vi "MegaAwesome_9_20_12a_JW.vi"() -> ()   [LabVIEW 2011]
uses:
  MegaAwesome_States.ctl
  <vilib>/Utility/file.llb/Read From Spreadsheet File (string).vi
  <vilib>/Utility/file.llb/Write To Spreadsheet File (string).vi
  <vilib>/Utility/inputDevices.llb/keyboardAcquire.vi
panel:
  in  "Slider Min":dbl=5.0
  in  "Slider Max":dbl=5.0
  out "Opj X Axis":string
  out "X Axis Display Type":string
  in  "Index-Sat":dbl=5.0
  in  "Index-Lin":dbl=5.0
  in  "IndexLog-Lin":dbl=5.0
  in  "IndexLog-Sat":dbl=5.0 caption="Num Pts"
  out "Lin Id-Log Used":dbl[](array[numeric])
  out "Lin-Vg Array-Log Used":dbl[](array[numeric])
  in  "New: Comments":string
  out "Save Array":string[][](array[string])
  out "Folder Index":i32 caption="Length"
  out "Sat Id-Used":dbl[](array[numeric])
  out "Sat Vg Array-Used":dbl[](array[numeric])
  out "Vg Array-Log-Used":dbl[](array[numeric])
  out "Sat Id-Log-Used":dbl[](array[numeric])
  out "Lin Id-Used":dbl[](array[numeric])
  out "Lin-Vg Array-Used":dbl[](array[numeric])
  out "Lin Vd":dbl
  out "Recorded Prop":T1
  out "Current State":T2
  in  "Main Tab Control":T3(tab)
  in  "Image Folder":path
  out "Image File":path=path "D:/UserData/Desktop/Jeremy/WFU/Research/Programs/VI mods/Image Not Found.png"
  in  "Transfer File":path
  out "Transfer Folder":path
  out "Fabrication Prop":T4
  in  "Transport ?":bool
  out "Distances":dbl[](array[numeric])
  in  "Zoom":i16(slide)=-3 scale=-5.0..5.0
  in  "Magnification":u16(ring) items=["5x", "10x", "20x", "50x", "80x"]
  in  "Undo Button":bool
  in  "Remove Button":bool
  in  "Transfer Plots":T5(tab)=enum."Saturation"
  in  "Lin-Trans Slider":dbl(slide) step=1.0 scale=-40.0..40.0 scale format="%#_1p"
  out "Sqrt-Lin":cluster{dbl[], dbl[]}[](graph)
  in  "Sat-Trans Slider":dbl(slide) step=1.0 scale=-40.0..40.0 scale format="%#_1p"
  out "Sqrt-Sat":cluster{dbl[], dbl[]}[](graph)
  out "Raw- Lin":cluster{dbl[], dbl[]}[](graph)
  out "Raw- Sat":cluster{dbl[], dbl[]}[](graph)
  in  "Log Plots":enum32{"Linear", "Saturation", "Transport"}(tab)=enum."Saturation"
  in  "Lin-Log Slider":dbl(slide) step=1.0 scale=-40.0..40.0 scale format="%#_1p"
  out "Log-Lin":cluster{dbl[], dbl[]}[](graph)
  in  "Sat-Log Slider":dbl(slide) step=1.0 scale=-40.0..40.0 scale format="%#_1p"
  out "Sat-Log":cluster{dbl[], dbl[]}[](graph)
  out "Transport":cluster{dbl[], dbl[]}[](graph)
  in  "Manual Controls":T6
  in  "File Controls":T7
  out "Date Recorded":string="Date Recorded" caption="Measured"
  out "Data Name:":string
  out "Image Name":string
  out "Index":string
  out "Date Created":string caption="Fabricated"
  in  "Comments:":string
  out "Rec: Length":dbl caption="Length" format="%#_3g"
  out "Rec: Width":dbl caption="Width" format="%#_4g"
  out "Rec: Dielectric (d)":dbl caption="Dielectric (d)" format="%#_3g"
  in  "New: Dielectric":dbl
  in  "New: Length":dbl
  in  "New: Width":dbl
  out "Rec: Temp":dbl caption="Sample Temp" format="%.1f"
  in  "New: Temp":dbl format="%.1f"
  out "Image Out":T8(plugin-control)
  in  "Num Pts":dbl=5.0
  in  "Num Pts Log":dbl=5.0 caption="Num Pts"
  out "Recorded Values Cluster":T9
  out "Calculated Values Cluster":T9 caption="Recorded Values Cluster"
  out "Re-Calculated Values Cluster":T9 caption="Recorded Values Cluster"
  in  "Independant Variable:":string(combo)="Length (um):"
  out "Image Preview":T8(plugin-control)
  out "Total Width":dbl
  in  "No Image File":path=path "\\\\acad1\\physics/Jurchescu-group/JW-PD/Mega Awesome/Image Not Found.png"
  in  "Room Temp":dbl=294.0
  in  "Origin Project File":path=path "\\\\acad1\\physics/Jurchescu-group/JW-PD/Group Library/Origin Project Files/DeviceData_8_10_12a_JW.opj"
  in  "Transport Style Controls":T10={"Transport Line Size"=1, "Transport Line Color"=16772608} {"Transport Line Size" items=["Extra Small", "Small", "Medium", "Large", "Extra Large"]}
  # "Image Location"
  # "Recorded"
  # "Calculated"
  # "Re-Calculated"
  # "Manual"
  # "Used points display at y=0\nValues are wrong w/ slider"
  # "Slider\nDoesn't\nWork"
  # "Slider\nDoesn't\nWork"
  # "No new points displayed"
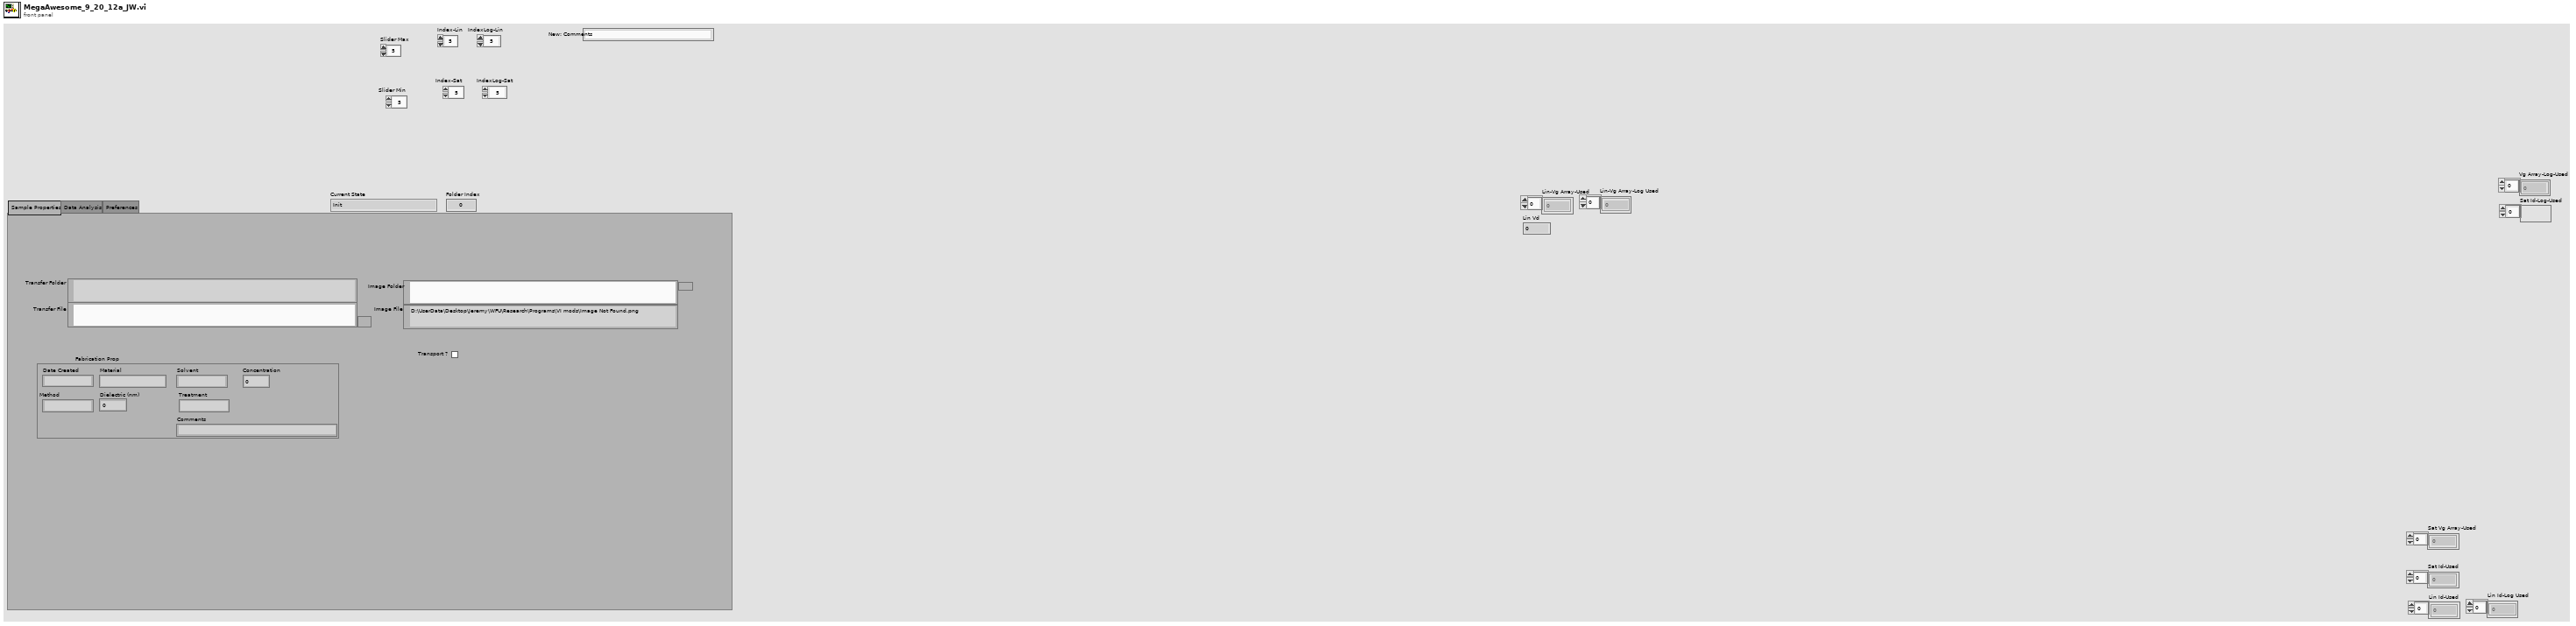
[diagram p1: front panel]
types:
  T1 = cluster{"Date Recorded":string, "Index":string, "Length":dbl, "Width":dbl, "Sample Temp":dbl}
  T2 = typedef "MegaAwesome_States.ctl" = enum16{"Init", "File Missing", "No Event", "Read Data", "Calculated Values", "Re-Calculated Values", "Next File", "Previous File", "Discard File", "Save", "Save Lines", "Export", "Exit"}
  T3 = enum32{"Sample Properties", "Data Analysis", "Preferences"}
  T4 = cluster{"Date Created":string, "Material":string, "Solvent":string, "Concentration":dbl, "Method":string, "Dielectric (nm)":dbl, "Treatment":string, "Comments":string}
  T5 = enum32{"Linear", "Saturation", "Raw-Linear", "Raw-Saturation"}
  T6 = cluster{"Manual-Temp":bool, "Manual-Width":bool, "Manuel-Length":bool, "Manuel-Dielectric":bool, "Manual Comments":bool}
  T7 = cluster{"Previous File":bool, "Discard ":bool, "Save Lines":bool, "Close":bool, "Next File ":bool, "Save":bool, "Save Next":bool, "Export":bool}
  T8 = typedef "IMAQ Image.ctl" = refnum<image>
  T9 = cluster{"Mobility-Sat":dbl, "Moblitity-Lin":dbl, "On/Off":dbl, "Off Current":dbl, "Vt-Sat":dbl, "STS":dbl, "Trap Density-VT":dbl, "Trap Density-STS":dbl}
  T10 = cluster{"Transport Line Size":u16, "Transport Line Color":u32}
  T11 = typedef "LVBoundsTypeDef.ctl" = cluster{"Width":u32, "Height":u32}
  T12 = enum16{"0", "1", "2", "3", "4", "5", "6", "7", "8", "9", "A", "B", "C", "D", "E", "F", "G", "H", "I", "J", "K", "L", "M", "N", "O", "P", "Q", "R", "S", "T", "U", "V", "W", "X", "Y", "Z", "F1", "F2", "F3", "F4", "F5", "F6", "F7", "F8", "F9", "F10", "F11", "F12", "F13", "F14", "F15", "ADD", "BACK", "BACKSLASH", "CAPITAL", "COMMA", "DECIMAL", "DELETE", "DIVIDE", "DOWN", "END", "EQUALS", "ESCAPE", "GRAVE (`)", "HOME", "INSERT", "LBRACKET", "LCONTROL", "LEFT", "L ALT", "LSHIFT", "LWIN", "MINUS", "MULTIPLY", "NEXT", "NUMLOCK", "NUMPAD_0", "NUMPAD_1", "NUMPAD_2", "NUMPAD_3", "NUMPAD_4", "NUMPAD_5", "NUMPAD_6", "NUMPAD_7", "NUMPAD_8", "NUMPAD_9", "PAUSE", "PERIOD", "PRIOR (PG UP)", "RBRACKET", "RCONTROL", "RETURN", "RIGHT", "R ALT", "RSHIFT", "RWIN", "SCROLL", "SEMICOLON", "SLASH", "SPACE", "SUBTRACT", "TAB", "UP", "ENTER (num pad)", "' (quote)"}[]
  T13 = enum16{"0", "1", "2", "3", "4", "5", "6", "7", "8", "9", "A", "B", "C", "D", "E", "F", "G", "H", "I", "J", "K", "L", "M", "N", "O", "P", "Q", "R", "S", "T", "U", "V", "W", "X", "Y", "Z", "F1", "F2", "F3", "F4", "F5", "F6", "F7", "F8", "F9", "F10", "F11", "F12", "F13", "F14", "F15", "ADD", "BACK", "BACKSLASH", "CAPITAL", "COMMA", "DECIMAL", "DELETE", "DIVIDE", "DOWN", "END", "EQUALS", "ESCAPE", "GRAVE (`)", "HOME", "INSERT", "LBRACKET", "LCONTROL", "LEFT", "L ALT", "LSHIFT", "LWIN", "MINUS", "MULTIPLY", "NEXT", "NUMLOCK", "NUMPAD_0", "NUMPAD_1", "NUMPAD_2", "NUMPAD_3", "NUMPAD_4", "NUMPAD_5", "NUMPAD_6", "NUMPAD_7", "NUMPAD_8", "NUMPAD_9", "PAUSE", "PERIOD", "PRIOR (PG UP)", "RBRACKET", "RCONTROL", "RETURN", "RIGHT", "R ALT", "RSHIFT", "RWIN", "SCROLL", "SEMICOLON", "SLASH", "SPACE", "SUBTRACT", "TAB", "UP", "ENTER (num pad)", "' (quote)"}
  T14 = typedef "ROI Descriptor" = cluster{"Global Rectangle":i32[], "Contours":cluster{"ID":enum32{"External", "Internal"}, "Type":u32, "Coordinates":i32[]}[]}
  T15 = cluster{string, sgl, bool, bool, bool, bool, bool, bool, i32}
  T16 = cluster{"[0]":cluster{dbl[], dbl[]}, "[1]":cluster{dbl[], dbl[]}, "[2]":cluster{dbl[], dbl[]}, "[3]":cluster{dbl[], dbl[]}, "[4]":cluster{dbl[], dbl[]}, "[5]":cluster{dbl[], dbl[]}, "[6]":cluster{dbl[], dbl[]}, "[7]":cluster{dbl[], dbl[]}, "[8]":cluster{dbl[], dbl[]}}
  T17 = cluster{"Sat Vg Used":dbl[], "Sat Sqrt(Id) Used ":dbl[], "Lin Vg Used":dbl[], "Lin Sqrt(Id) Used":dbl[], "Index-Lin":dbl, "Index-Sat":dbl}
  T18 = cluster{"Raw Sat":cluster{dbl[], dbl[]}[], "Sqrt Sat":cluster{dbl[], dbl[]}[], "Log Sat":cluster{dbl[], dbl[]}[], "Raw Lin":cluster{dbl[], dbl[]}[], "Sqrt Lin":cluster{dbl[], dbl[]}[], "Log Lin":cluster{dbl[], dbl[]}[]}
  T19 = cluster{"Mobility-Sat":dbl, "Vt-Sat":dbl, "Mobility-Lin":dbl, "Vt-Lin":dbl, "Off I-Sat":dbl, "On/Off I-Sat":dbl}
  T20 = cluster{"Sat Vg Used":dbl[], "Sat Log(Id) Used":dbl[], "Lin Vg Used":dbl[], "Lin Log(Id) Used":dbl[], "STS Index-Sat":dbl, "STS Index-Lin":dbl}
  T21 = cluster{"Independant  Variable Indicator":string, "Parameter String Indicator":string}
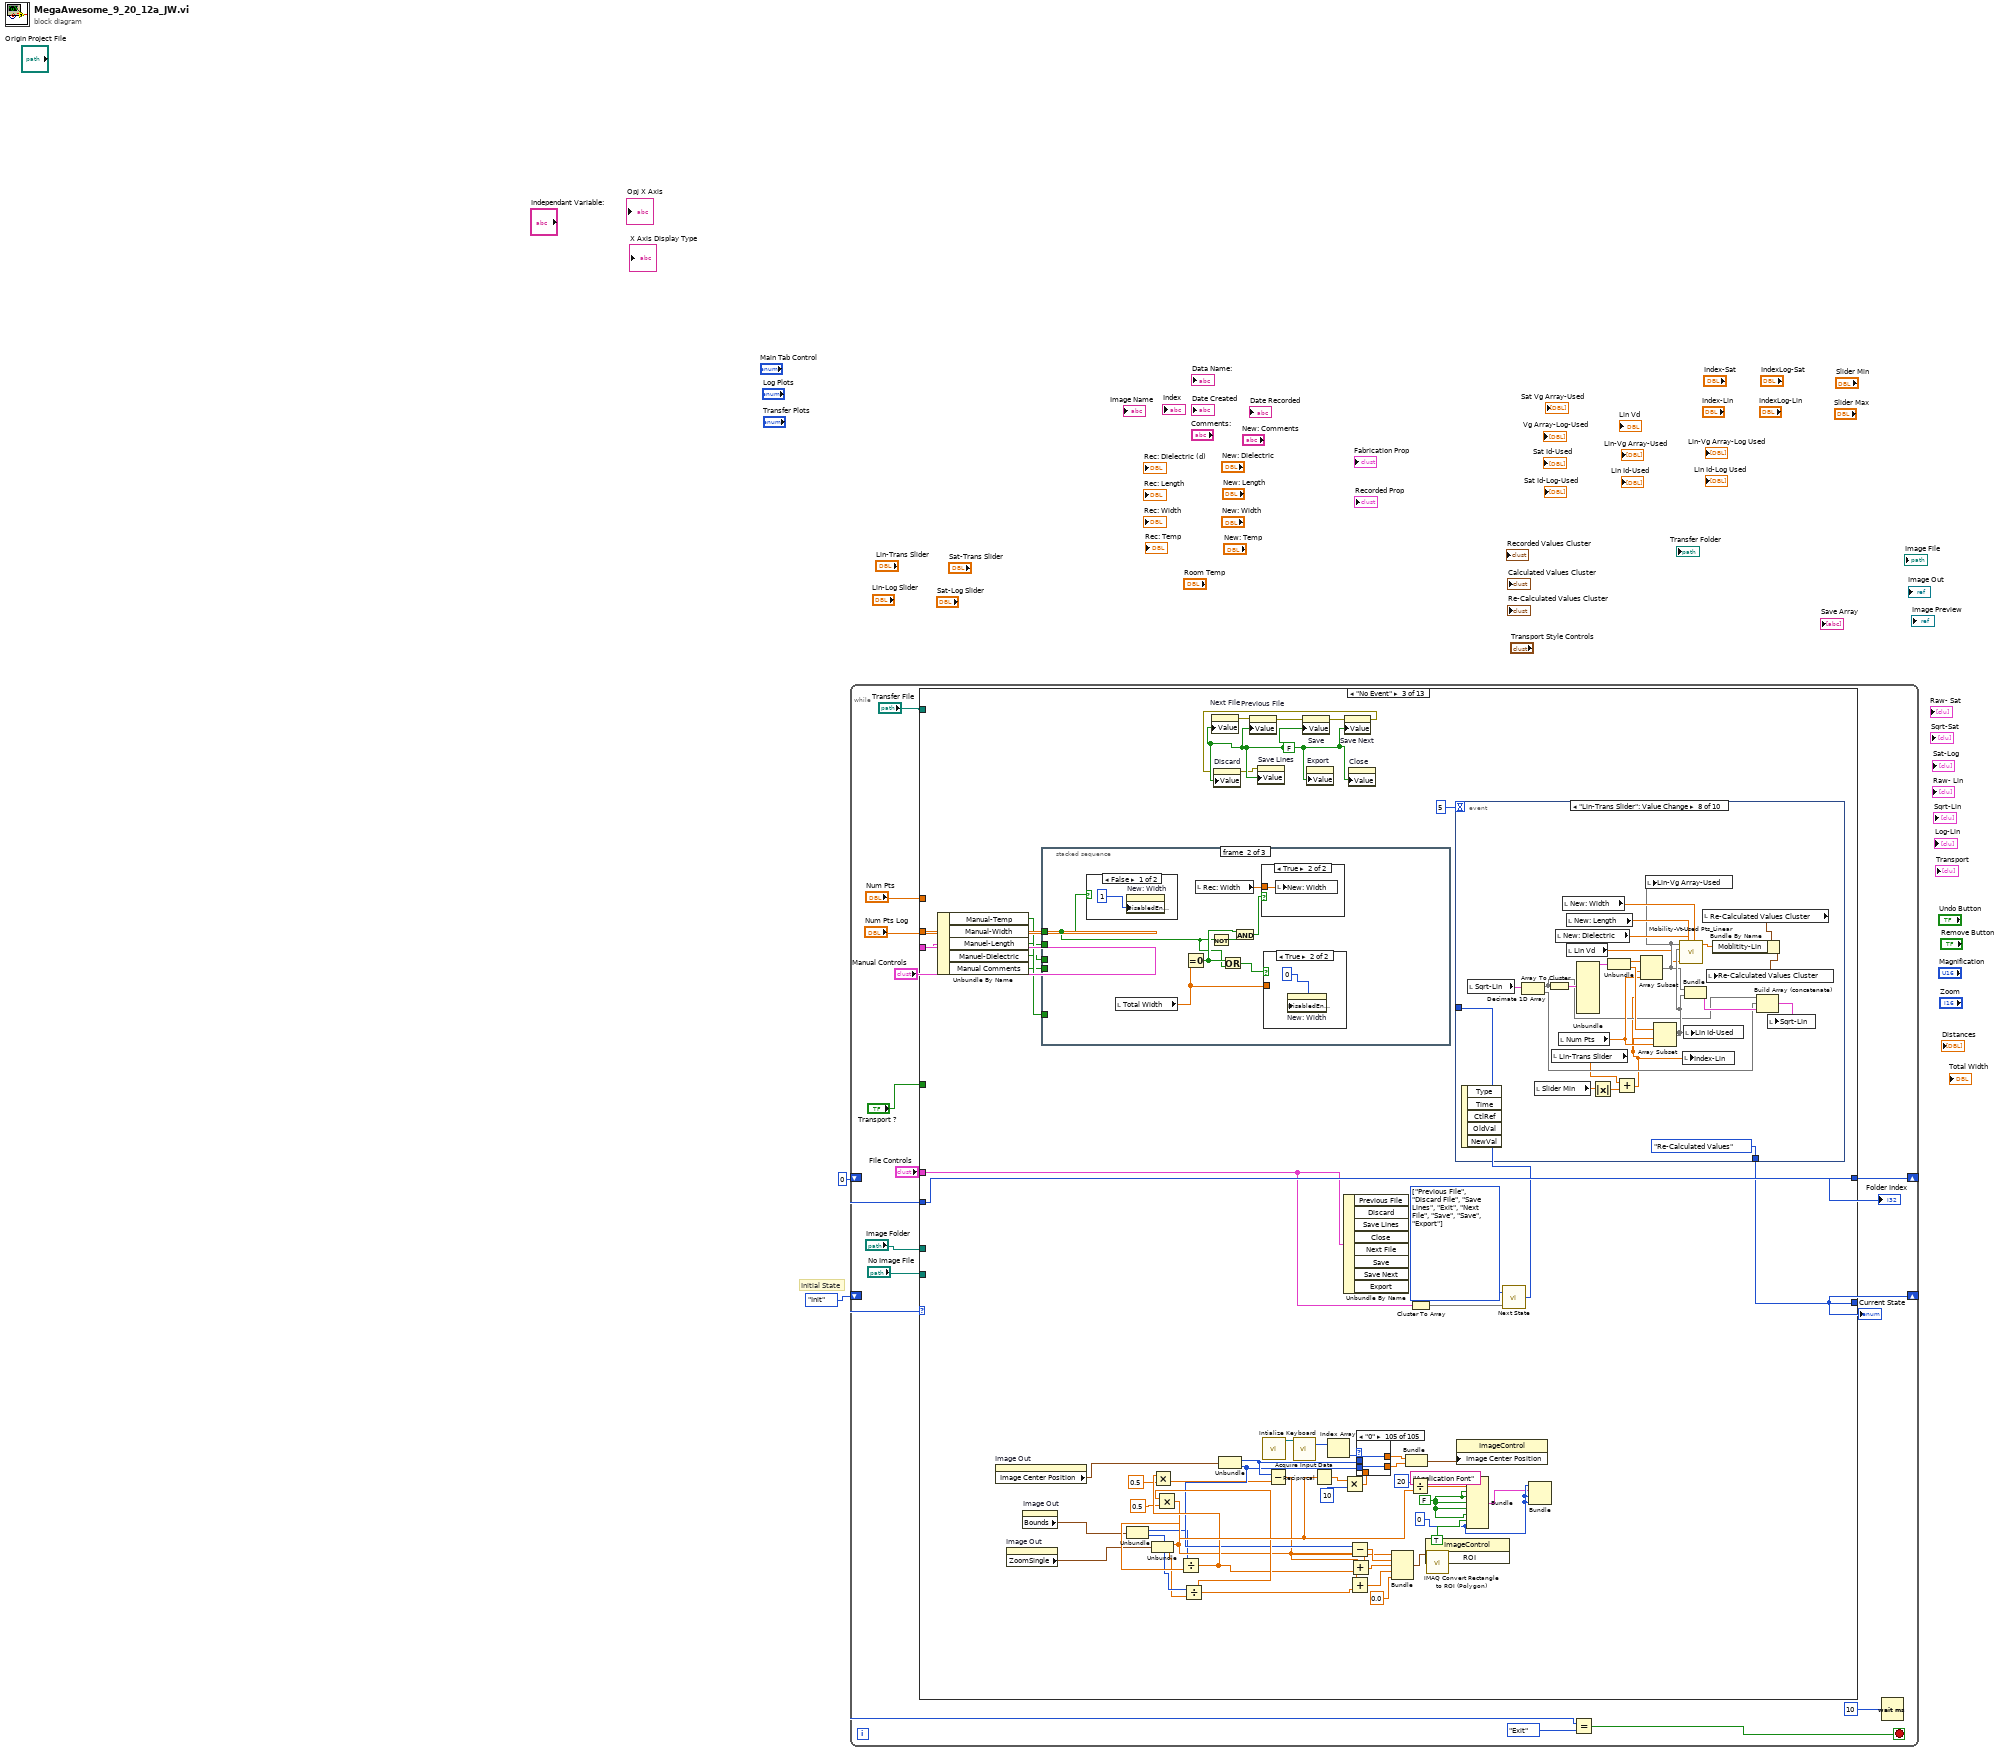
[diagram p0: block diagram]
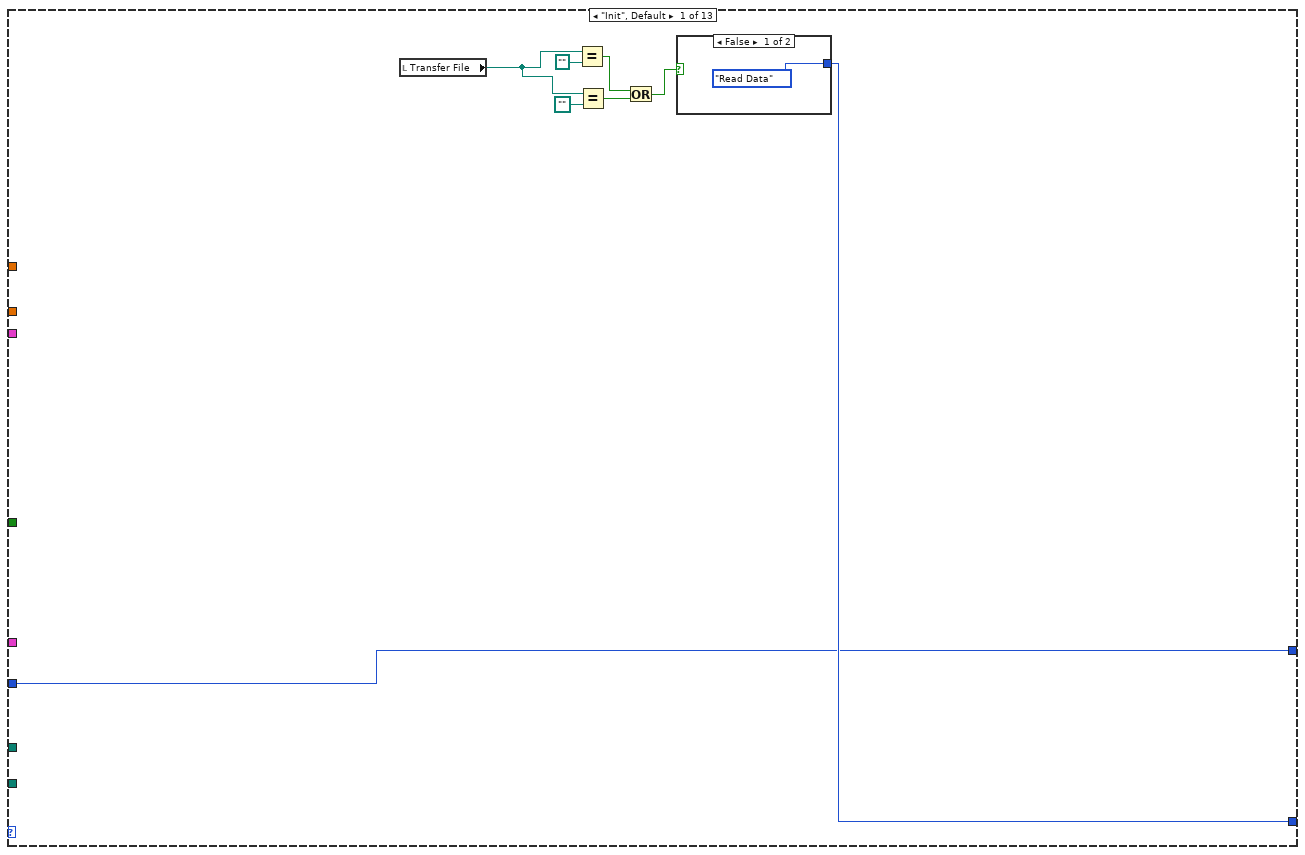
[diagram p2: hidden frame]
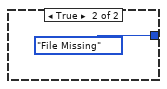
[diagram p3: hidden frame]
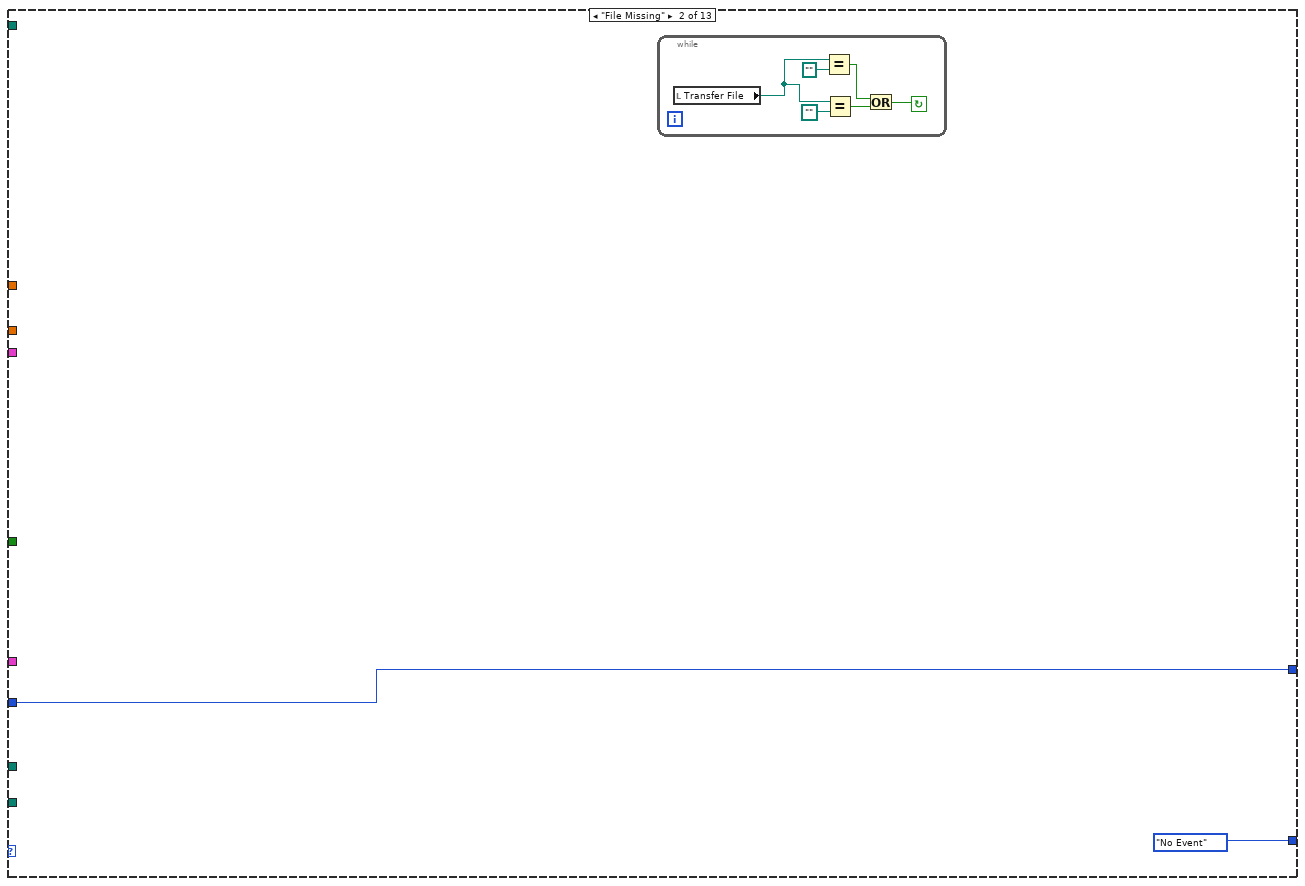
[diagram p4: hidden frame]
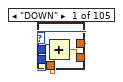
[diagram p5: hidden frame]
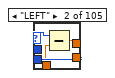
[diagram p6: hidden frame]
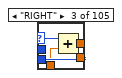
[diagram p7: hidden frame]
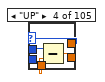
[diagram p8: hidden frame]
diagram:
  # "Initial State"
  n1 = while {
    shift-right: [w14] -> _
    shift-left: MegaAwesome_States."Init" -> [w16]
    shift-right: [w7] -> _
    shift-left: 0 -> [w8]
    stop <- w17 stop-if-true
    n2 = case shown="\"No Event\"" w16 {
      tunnel: [w19 MegaAwesome_States."No Event" w82 MegaAwesome_States."Calculated Values" MegaAwesome_States."Re-Calculated Values" MegaAwesome_States."No Event" MegaAwesome_States."Read Data" MegaAwesome_States."Read Data" MegaAwesome_States."No Event" w600 MegaAwesome_States."No Event" MegaAwesome_States."No Event" MegaAwesome_States."Exit"] -> w14
      tunnel: "Transfer File" -> [_ _ _ w445 w480 _ w569 w581 _ w605 _ _ _]
      tunnel: "Num Pts" -> [_ _ _ _ w504 _ _ _ _ _ _ _ _]
      tunnel: "Num Pts Log" -> [_ _ _ _ w503 _ _ _ _ _ _ _ _]
      tunnel: "Image Folder" -> [_ _ _ _ w500 _ _ _ _ _ _ _ _]
      tunnel: "No Image File" -> [_ _ _ _ w499 _ _ _ _ _ _ _ _]
      tunnel: [w18 w28 w90 w439 w498 w529 w554 w579 w597 w606 w1121 w1124 w1125] -> w7
      tunnel: w8 -> [w18 w28 w90 _ w498 w529 w555 w580 w597 w606 w1121 w1124 w1125]
      tunnel: "Manual Controls" -> [_ _ w84 _ _ _ _ _ _ w604 _ _ _]
      tunnel: "File Controls" -> [_ _ w80 _ _ _ _ _ _ w599 _ _ _]
      tunnel: "Transport ?" -> [_ _ _ _ w466 _ _ _ _ _ _ _ _]
      frame "Init", Default {
        n3 = local read "Transfer File"() -> (w20:path)
        n4 = Equal?(x=w20, y=path "") -> (x = y?=w23:bool)
        n5 = Equal?(x=w20, y=path "") -> (x = y?=w22:bool)
        n6 = Or(x=w23, y=w22) -> (x .or. y?=w25:bool)
        n7 = case shown="False" w25 {
          tunnel: [MegaAwesome_States."Read Data" MegaAwesome_States."File Missing"] -> w19
          frame False {
          }
          frame True {
          }
        }
      }
      frame "File Missing" {
        n8 = while {
          stop <- w30 continue-if-true
          n9 = local read "Transfer File"() -> (w31:path)
          n10 = Equal?(x=w31, y=path "") -> (x = y?=w33:bool)
          n11 = Equal?(x=w31, y=path "") -> (x = y?=w34:bool)
          n12 = Or(x=w33, y=w34) -> (x .or. y?=w30:bool)
        }
      }
      frame "No Event" {
        w64 = FALSE
        w66 = 0
        w79 = FALSE
        w92 = T2[] [enum."Previous File", enum."Discard File", enum."Save Lines", enum."Exit", enum."Next File", enum."Save", enum."Save", enum."Export"] items=["Init", "File Missing", "No Event", "Read Data", "Calculated Values", "Re-Calculated Values", "Next File", "Previous File", "Discard File", "Save", "Save Lines", "Export", "Exit"]
        n13 = Unbundle By Name(w84) -> ("Manual-Temp"=w89:bool, "Manual-Width"=w88:bool, "Manuel-Length"=w87:bool, "Manuel-Dielectric"=w86:bool, "Manual Comments"=w85:bool)
        n14 = property on="Image Out" class="ImageControl"() -> ("Image Center Position"=w42:cluster{"X":u32, "Y":u32})  [unwired: 2 in, 2 out]
        n15 = property on="Image Out" class="ImageControl"() -> ("ZoomSingle"=w49:cluster{"X":sgl, "Y":sgl})  [unwired: 2 in, 2 out]
        n16 = property on="Image Out" class="ImageControl"() -> ("Bounds"=w48:T11)  [unwired: 2 in, 2 out]
        n17 = stacked-sequence {
          tunnel: w89 -> [w403 _ _]
          tunnel: w88 -> [_ w413 _]
          tunnel: w87 -> [_ _ w428]
          tunnel: w86 -> [_ _ w425]
          tunnel: w85 -> [_ _ w424]
          frame #0 {
            n18 = local read "Rec: Temp"() -> (w402:dbl)
            n19 = case shown="False" w403 {
              tunnel: w402 -> [w408 _]
              tunnel: [w405 w412] -> _
              frame False {
                n20 = local read "Rec: Temp"() -> (w406:dbl)
                n21 = property on="New: Temp" class="DigNum (strict)"("DisabledEnum"=1) -> ()  [unwired: 2 in, 2 out]
                n22 = Equal To 0?(x=w406) -> (x = 0?=w407:bool)
                n23 = local write "New: Temp"(w408) -> ()
                n24 = case shown="True" w407 {
                  tunnel: [w409 w410] -> w405
                  tunnel: w406 -> [w409 _]
                  frame False {
                  }
                  frame True {
                    n25 = local read "Room Temp"() -> (w410:dbl)
                  }
                }
                n26 = local write "New: Temp"(w405) -> ()
              }
              frame True {
                n27 = property on="New: Temp" class="DigNum (strict)"("DisabledEnum"=0) -> ()  [unwired: 2 in, 2 out]
                n28 = local read "New: Temp"() -> (w412:dbl)
              }
            }
          }
          frame #1 {
            n29 = case shown="False" w413 {
              frame False {
                n30 = property on="New: Width" class="DigNum (strict)"("DisabledEnum"=1) -> ()  [unwired: 2 in, 2 out]
              }
              frame True {
                (unwired) 0
              }
            }
            n31 = local read "Total Width"() -> (w419:dbl)
            n32 = Equal To 0?(x=w419) -> (x = 0?=w416:bool)
            n33 = local read "Rec: Width"() -> (w417:dbl)
            n34 = Not(x=w413) -> (.not. x?=w415:bool)
            n35 = Or(x=w416, y=w413) -> (x .or. y?=w418:bool)
            n36 = And(x=w416, y=w415) -> (x .and. y?=w414:bool)
            n37 = case shown="True" w414 {
              tunnel: w417 -> [_ w421]
              frame False {
              }
              frame True {
                n38 = local write "New: Width"(w421) -> ()
              }
            }
            n39 = case shown="True" w418 {
              tunnel: w419 -> [w422 _]
              frame False {
                (unwired) 1
                n40 = local write "New: Width"(w422) -> ()
              }
              frame True {
                n41 = property on="New: Width" class="DigNum (strict)"("DisabledEnum"=0) -> ()  [unwired: 2 in, 2 out]
              }
            }
          }
          frame #2 {
            n42 = local read "Rec: Length"() -> (w429:dbl)
            n43 = case shown="True" w428 {
              tunnel: w429 -> [w437 _]
              frame False {
                n44 = local write "New: Length"(w437) -> ()
                n45 = property on="New: Length" class="DigNum (strict)"("DisabledEnum"=1) -> ()  [unwired: 2 in, 2 out]
              }
              frame True {
                n46 = property on="New: Length" class="DigNum (strict)"("DisabledEnum"=0) -> ()  [unwired: 2 in, 2 out]
              }
            }
            n47 = local read "Comments:"() -> (w426:string)
            n48 = local read "Rec: Dielectric (d)"() -> (w427:dbl)
            n49 = case shown="True" w424 {
              tunnel: w426 -> [w431 _]
              frame False {
                n50 = local write "New: Comments"(w431) -> ()
                n51 = property on="New: Comments" class="Str"("DisabledEnum"=1) -> ()  [unwired: 2 in, 2 out]
              }
              frame True {
                n52 = property on="New: Comments" class="Str"("DisabledEnum"=0) -> ()  [unwired: 2 in, 2 out]
              }
            }
            n53 = case shown="True" w425 {
              tunnel: w427 -> [w434 _]
              frame False {
                n54 = local write "New: Dielectric"(w434) -> ()
                n55 = property on="New: Dielectric" class="DigNum (strict)"("DisabledEnum"=1) -> ()  [unwired: 2 in, 2 out]
              }
              frame True {
                n56 = property on="New: Dielectric" class="DigNum (strict)"("DisabledEnum"=0) -> ()  [unwired: 2 in, 2 out]
              }
            }
          }
        }
        n57 = Unbundle(w48) -> ("Width"=w51:u32, "Height"=w52:u32)
        n58 = Unbundle(w49) -> ("X"=w71:sgl, "Y"=w50:sgl)
        n59 = Divide(x=w51, y=w71) -> (x/y=w61:sgl)
        n60 = Multiply(x=w61, y=0.5) -> (x*y=w55:dbl)
        n61 = Divide(x=w52, y=w50) -> (x/y=w62:sgl)
        n62 = Multiply(x=w62, y=0.5) -> (x*y=w56:dbl)
        n63 = property on="Next File" class="Bool (strict)"("Value"=w79) -> (error out=w78:errorcluster)  [unwired: 2 in, 1 out]
        n64 = Unbundle(w42) -> ("X"=w60:u32, "Y"=w59:u32)
        n65 = property on="Previous File" class="Bool (strict)"(error in=w78, "Value"=w79) -> (error out=w77:errorcluster)  [unwired: 1 in, 1 out]
        n66 = call <vilib>:"Intialize Keyboard.vi"() -> ("device ID"=w39:refnum<k1>)  [unwired: 10 in, 1 out]
        n67 = Subtract(x=w60, y=w55) -> (x-y=w57:dbl)
        n68 = call-poly <vilib>:"Acquire Input Data.vi"("device ID"=w39) -> ("keys pressed"=w40:T12)  [unwired: 16 in, 2 out]
        n69 = property on="Save" class="Bool (strict)"(error in=w77, "Value"=w79) -> (error out=w76:errorcluster)  [unwired: 1 in, 1 out]
        n70 = property on="Export" class="Bool (strict)"("Value"=w79) -> ()  [unwired: 2 in, 2 out]
        n71 = Reciprocal(x=w71) -> (1/x=w72:sgl)
        n72 = Index Array(array=w40) -> (element=w36:T13)  [unwired: 1 in]
        n73 = Unbundle By Name(w80) -> ()  [unwired: 8 out]
        n74 = Multiply(x=w72, y=10) -> (x*y=w70:sgl)
        n75 = property on="Save Next" class="Bool (strict)"(error in=w76, "Value"=w79) -> (error out=w75:errorcluster)  [unwired: 1 in, 1 out]
        n76 = property on="Discard" class="Bool (strict)"(error in=w75, "Value"=w79) -> (error out=w74:errorcluster)  [unwired: 1 in, 1 out]
        n77 = property on="Save Lines" class="Bool (strict)"(error in=w74, "Value"=w79) -> ()  [unwired: 1 in, 2 out]
        n78 = property on="Close" class="Bool (strict)"("Value"=w79) -> ()  [unwired: 2 in, 2 out]
        n79 = Subtract(x=w59, y=w56) -> (x-y=w58:dbl)
        n80 = Add(x=w58, y=w62) -> (x+y=w44:dbl)
        n81 = Add(x=w57, y=w61) -> (x+y=w43:dbl)
        n82 = case shown="\"0\"" w36 {
          tunnel: w60 -> [w94 w100 w104 w106 w110 w112 w114 w116 w118 w120 w122 w124 w126 w128 w130 w132 w134 w136 w138 w140 w142 w144 w146 w148 w150 w152 w154 w156 w158 w160 w162 w164 w166 w168 w170 w172 w174 w176 w178 w180 w182 w184 w186 w188 w190 w192 w194 w196 w198 w200 w202 w204 w206 w208 w210 w212 w214 w216 w218 w220 w222 w224 w226 w228 w230 w232 w234 w236 w238 w240 w242 w244 w246 w248 w250 w252 w254 w256 w258 w260 w262 w264 w266 w268 w270 w272 w274 w276 w278 w280 w282 w284 w286 w288 w290 w292 w294 w296 w298 w300 w302 w304 w306 w308 w310]
          tunnel: [w94 w99 w103 w106 w110 w112 w114 w116 w118 w120 w122 w124 w126 w128 w130 w132 w134 w136 w138 w140 w142 w144 w146 w148 w150 w152 w154 w156 w158 w160 w162 w164 w166 w168 w170 w172 w174 w176 w178 w180 w182 w184 w186 w188 w190 w192 w194 w196 w198 w200 w202 w204 w206 w208 w210 w212 w214 w216 w218 w220 w222 w224 w226 w228 w230 w232 w234 w236 w238 w240 w242 w244 w246 w248 w250 w252 w254 w256 w258 w260 w262 w264 w266 w268 w270 w272 w274 w276 w278 w280 w282 w284 w286 w288 w290 w292 w294 w296 w298 w300 w302 w304 w306 w308 w310] -> w37
          tunnel: w59 -> [w96 w98 w102 w108 w109 w111 w113 w115 w117 w119 w121 w123 w125 w127 w129 w131 w133 w135 w137 w139 w141 w143 w145 w147 w149 w151 w153 w155 w157 w159 w161 w163 w165 w167 w169 w171 w173 w175 w177 w179 w181 w183 w185 w187 w189 w191 w193 w195 w197 w199 w201 w203 w205 w207 w209 w211 w213 w215 w217 w219 w221 w223 w225 w227 w229 w231 w233 w235 w237 w239 w241 w243 w245 w247 w249 w251 w253 w255 w257 w259 w261 w263 w265 w267 w269 w271 w273 w275 w277 w279 w281 w283 w285 w287 w289 w291 w293 w295 w297 w299 w301 w303 w305 w307 w309]
          tunnel: [w95 w98 w102 w107 w109 w111 w113 w115 w117 w119 w121 w123 w125 w127 w129 w131 w133 w135 w137 w139 w141 w143 w145 w147 w149 w151 w153 w155 w157 w159 w161 w163 w165 w167 w169 w171 w173 w175 w177 w179 w181 w183 w185 w187 w189 w191 w193 w195 w197 w199 w201 w203 w205 w207 w209 w211 w213 w215 w217 w219 w221 w223 w225 w227 w229 w231 w233 w235 w237 w239 w241 w243 w245 w247 w249 w251 w253 w255 w257 w259 w261 w263 w265 w267 w269 w271 w273 w275 w277 w279 w281 w283 w285 w287 w289 w291 w293 w295 w297 w299 w301 w303 w305 w307 w309] -> w38
          tunnel: w70 -> [w93 w97 w101 w105 _ _ _ _ _ _ _ _ _ _ _ _ _ _ _ _ _ _ _ _ _ _ _ _ _ _ _ _ _ _ _ _ _ _ _ _ _ _ _ _ _ _ _ _ _ _ _ _ _ _ _ _ _ _ _ _ _ _ _ _ _ _ _ _ _ _ _ _ _ _ _ _ _ _ _ _ _ _ _ _ _ _ _ _ _ _ _ _ _ _ _ _ _ _ _ _ _ _ _ _ _]
          frame "DOWN" {
            n83 = Add(x=w96, y=w93) -> (x+y=w95:sgl)
          }
          frame "LEFT" {
            n84 = Subtract(x=w100, y=w97) -> (x-y=w99:sgl)
          }
          frame "RIGHT" {
            n85 = Add(x=w104, y=w101) -> (x+y=w103:sgl)
          }
          frame "UP" {
            n86 = Subtract(x=w108, y=w105) -> (x-y=w107:sgl)
          }
          frame "ENTER (num pad)" {
          }
          frame "' (quote)" {
          }
          frame "END" {
          }
          frame "EQUALS" {
          }
          frame "ESCAPE" {
          }
          frame "GRAVE (`)" {
          }
          frame "HOME" {
          }
          frame "INSERT" {
          }
          frame "LBRACKET" {
          }
          frame "LCONTROL" {
          }
          frame "L ALT" {
          }
          frame "LSHIFT" {
          }
          frame "LWIN" {
          }
          frame "MINUS" {
          }
          frame "MULTIPLY" {
          }
          frame "NEXT" {
          }
          frame "NUMLOCK" {
          }
          frame "NUMPAD_0" {
          }
          frame "NUMPAD_1" {
          }
          frame "NUMPAD_2" {
          }
          frame "NUMPAD_3" {
          }
          frame "NUMPAD_4" {
          }
          frame "NUMPAD_5" {
          }
          frame "NUMPAD_6" {
          }
          frame "NUMPAD_7" {
          }
          frame "NUMPAD_8" {
          }
          frame "NUMPAD_9" {
          }
          frame "PAUSE" {
          }
          frame "PERIOD" {
          }
          frame "PRIOR (PG UP)" {
          }
          frame "RBRACKET" {
          }
          frame "RCONTROL" {
          }
          frame "RETURN" {
          }
          frame "R ALT" {
          }
          frame "RSHIFT" {
          }
          frame "RWIN" {
          }
          frame "SCROLL" {
          }
          frame "SEMICOLON" {
          }
          frame "SLASH" {
          }
          frame "SPACE" {
          }
          frame "SUBTRACT" {
          }
          frame "TAB" {
          }
          frame "DIVIDE" {
          }
          frame "DELETE" {
          }
          frame "DECIMAL" {
          }
          frame "COMMA" {
          }
          frame "CAPITAL" {
          }
          frame "BACKSLASH" {
          }
          frame "BACK" {
          }
          frame "ADD" {
          }
          frame "F15" {
          }
          frame "F14" {
          }
          frame "F13" {
          }
          frame "F12" {
          }
          frame "F11" {
          }
          frame "F10" {
          }
          frame "F9" {
          }
          frame "F8" {
          }
          frame "F7" {
          }
          frame "F6" {
          }
          frame "F5" {
          }
          frame "F4" {
          }
          frame "F3" {
          }
          frame "F2" {
          }
          frame "F1" {
          }
          frame "Z" {
          }
          frame "Y" {
          }
          frame "X" {
          }
          frame "W" {
          }
          frame "V" {
          }
          frame "U" {
          }
          frame "T" {
          }
          frame "S" {
          }
          frame "R" {
          }
          frame "Q" {
          }
          frame "P" {
          }
          frame "O" {
          }
          frame "N" {
          }
          frame "M" {
          }
          frame "L" {
          }
          frame "K" {
          }
          frame "J" {
          }
          frame "I" {
          }
          frame "H" {
          }
          frame "G" {
          }
          frame "F" {
          }
          frame "E" {
          }
          frame "D" {
          }
          frame "C" {
          }
          frame "B" {
          }
          frame "A" {
          }
          frame "9" {
          }
          frame "8" {
          }
          frame "7" {
          }
          frame "6" {
          }
          frame "5" {
          }
          frame "4" {
          }
          frame "3" {
          }
          frame "2" {
          }
          frame "1" {
          }
          frame "0" {
          }
        }
        n87 = Bundle(w57, w58, w43, w44, 0.0) -> (w45:cluster{dbl, dbl, dbl, dbl, dbl})  [unwired: 1 in]
        n88 = Bundle("X"=w37, "Y"=w38) -> (w41:cluster{"X":sgl, "Y":sgl})  [unwired: 1 in]
        n89 = Divide(x=20, y=w71) -> (x/y=w68:sgl)
        n90 = Cluster To Array(cluster=w80) -> (array=w91:bool[])
        n91 = call "IMAQ Convert Rectangle to ROI (Polygon)"("Rectangle"=w45) -> ("ROI Descriptor"=w47:T14)  [unwired: 7 in, 2 out]
        n92 = property on="Property Node" class="ImageControl"("ROI"=w47) -> ()  [unwired: 2 in, 2 out]
        n93 = property on="Property Node" class="ImageControl"("Image Center Position"=w41) -> ()  [unwired: 2 in, 2 out]
        n94 = Bundle("Application Font", w68, w64, w64, w64, w64, w64, TRUE, w66) -> (w63:T15)  [unwired: 1 in]
        n95 = call "Next State.vi"("Buttons []"=w91, "States []"=w92) -> ("Enum"=w83:T2)
        n96 = event shown="[7] \"Lin-Trans Slider\": Value Change" {
          selector: _ -> [_ _ _ _ _ _ _ _ _ _]
          dyn-events: _ -> [_ _ _ _ _ _ _ _ _ _]
          timeout: 5 -> [_ _ _ _ _ _ _ _ _ _]
          tunnel: w83 -> [w311 _ _ _ _ _ _ _ _ _]
          tunnel: [w311 MegaAwesome_States."Re-Calculated Values" MegaAwesome_States."Re-Calculated Values" MegaAwesome_States."Re-Calculated Values" MegaAwesome_States."Re-Calculated Values" MegaAwesome_States."Calculated Values" MegaAwesome_States."Re-Calculated Values" MegaAwesome_States."Re-Calculated Values" MegaAwesome_States."Re-Calculated Values" MegaAwesome_States."Re-Calculated Values"] -> w82
          event Timeout {
            n97 = event-data() -> ()  [unwired: 1 in, 2 out]
          }
          event "New: Dielectric": Value Change {
            n98 = event-data() -> ()  [unwired: 1 in, 5 out]
          }
          event "New: Length": Value Change {
            n99 = event-data() -> ()  [unwired: 1 in, 5 out]
          }
          event "New: Width": Value Change {
            n100 = event-data() -> ()  [unwired: 1 in, 5 out]
          }
          event "New: Temp": Value Change {
            n101 = event-data() -> ()  [unwired: 1 in, 5 out]
          }
          event "Num Pts Log", "Transport Style Controls", "Num Pts": Value Change {
            n102 = event-data() -> ()  [unwired: 1 in, 5 out]
          }
          event "Sat-Trans Slider": Value Change {
            n103 = event-data() -> ()  [unwired: 1 in, 5 out]
            n104 = local read "Sqrt-Sat"() -> (w340:cluster{dbl[], dbl[]}[])
            n105 = Decimate 1D Array(w340) -> (w324:cluster{dbl[], dbl[]}[], w325:cluster{dbl[], dbl[]}[])
            n106 = local read "Slider Min"() -> (w321:dbl)
            n107 = local read "Sat-Trans Slider"() -> (w319:dbl)
            n108 = Array To Cluster(array=w324) -> (cluster=w339:T16)
            n109 = local read "New: Dielectric"() -> (w334:dbl)
            n110 = local read "Num Pts"() -> (w317:dbl)
            n111 = local read "New: Width"() -> (w336:dbl)
            n112 = local read "New: Length"() -> (w335:dbl)
            n113 = Unbundle(w339) -> ("[0]"=w338:cluster{dbl[], dbl[]})  [unwired: 8 out]
            n114 = Absolute Value(x=w321) -> (abs(x)=w320:dbl)
            n115 = Unbundle(w338) -> (w322:dbl[], w337:dbl[])
            n116 = Add(x=w319, y=w320) -> (x+y=w318:dbl)
            n117 = Array Subset(array=w322, index=w318, length=w317) -> (w332:dbl[])
            n118 = local write "Sat Vg Array-Used"(w332) -> ()
            n119 = Array Subset(array=w337, index=w318, length=w317) -> (w333:dbl[])
            n120 = call "Mobility-Vt-Used Pts_Saturation.vi"("Width"=w336, "Length"=w335, "Dielectric (d)"=w334, "Sat Id Used"=w333, "Vg Used"=w332) -> ("Vt"=w328:dbl, "Mobility"=w329:dbl)  [unwired: 4 in, 1 out]
            n121 = local write "Index-Sat"(w318) -> ()
            n122 = local write "Sat Id-Used"(w333) -> ()
            n123 = Bundle(w332, w333) -> (w326:cluster{dbl[], dbl[]})  [unwired: 1 in]
            n124 = local read "Re-Calculated Values Cluster"() -> (w331:T9)
            n125 = Bundle By Name(cluster=w331, "Mobility-Sat"=w329, "Vt-Sat"=w328) -> (w330:T9)
            n126 = local write "Re-Calculated Values Cluster"(w330) -> ()
            n127 = Build Array (concatenate)(w324, w325, w326) -> (w323:cluster{dbl[], dbl[]}[])
            n128 = local write "Sqrt-Sat"(w323) -> ()
          }
          event "Lin-Trans Slider": Value Change {
            n129 = event-data() -> ()  [unwired: 1 in, 5 out]
            n130 = local read "Sqrt-Lin"() -> (w364:cluster{dbl[], dbl[]}[])
            n131 = Decimate 1D Array(w364) -> (w349:cluster{dbl[], dbl[]}[], w350:cluster{dbl[], dbl[]}[])
            n132 = local read "Slider Min"() -> (w346:dbl)
            n133 = Array To Cluster(array=w349) -> (cluster=w363:T16)
            n134 = local read "Lin-Trans Slider"() -> (w344:dbl)
            n135 = local read "New: Dielectric"() -> (w357:dbl)
            n136 = local read "Num Pts"() -> (w360:dbl)
            n137 = local read "New: Width"() -> (w359:dbl)
            n138 = local read "New: Length"() -> (w358:dbl)
            n139 = local read "Lin Vd"() -> (w341:dbl)
            n140 = Unbundle(w363) -> ("[0]"=w362:cluster{dbl[], dbl[]})  [unwired: 8 out]
            n141 = Absolute Value(x=w346) -> (abs(x)=w345:dbl)
            n142 = Unbundle(w362) -> (w347:dbl[], w361:dbl[])
            n143 = Add(x=w344, y=w345) -> (x+y=w343:dbl)
            n144 = Array Subset(array=w347, index=w343, length=w360) -> (w355:dbl[])
            n145 = local write "Lin-Vg Array-Used"(w355) -> ()
            n146 = Array Subset(array=w361, index=w343, length=w360) -> (w356:dbl[])
            n147 = call "Mobility-Vt-Used Pts_Linear.vi"("Width"=w359, "Length"=w358, "Vd"=w341, "Dielectric (d)"=w357, "Id Used"=w356, "Vg Used"=w355) -> ("Mobility"=w352:dbl)  [unwired: 3 in, 2 out]
            n148 = local write "Index-Lin"(w343) -> ()
            n149 = local write "Lin Id-Used"(w356) -> ()
            n150 = Bundle(w355, w356) -> (w351:cluster{dbl[], dbl[]})  [unwired: 1 in]
            n151 = local read "Re-Calculated Values Cluster"() -> (w354:T9)
            n152 = Bundle By Name(cluster=w354, "Moblitity-Lin"=w352) -> (w353:T9)
            n153 = local write "Re-Calculated Values Cluster"(w353) -> ()
            n154 = Build Array (concatenate)(w349, w350, w351) -> (w348:cluster{dbl[], dbl[]}[])
            n155 = local write "Sqrt-Lin"(w348) -> ()
          }
          event "Sat-Log Slider": Value Change {
            n156 = event-data() -> ()  [unwired: 1 in, 5 out]
            n157 = local read "Sat-Log"() -> (w367:cluster{dbl[], dbl[]}[])
            n158 = Decimate 1D Array(w367) -> (w374:cluster{dbl[], dbl[]}[], w375:cluster{dbl[], dbl[]}[])
            n159 = local read "Slider Min"() -> (w371:dbl)
            n160 = Array To Cluster(array=w374) -> (cluster=w384:T16)
            n161 = local read "Num Pts Log"() -> (w381:dbl)
            n162 = local read "Sat-Log Slider"() -> (w369:dbl)
            n163 = Unbundle(w384) -> ("[0]"=w383:cluster{dbl[], dbl[]})  [unwired: 8 out]
            n164 = Absolute Value(x=w371) -> (abs(x)=w370:dbl)
            n165 = Unbundle(w383) -> (w372:dbl[], w382:dbl[])
            n166 = Add(x=w369, y=w370) -> (x+y=w366:dbl)
            n167 = Array Subset(array=w372, index=w366, length=w381) -> (w379:dbl[])
            n168 = Array Subset(array=w382, index=w366, length=w381) -> (w380:dbl[])
            n169 = local write "Vg Array-Log-Used"(w379) -> ()
            n170 = local write "IndexLog-Sat"(w366) -> ()
            n171 = Bundle(w379, w380) -> (w365:cluster{dbl[], dbl[]})  [unwired: 1 in]
            n172 = call "STS-Used.vi"("Id Used"=w380, "Vg-Used"=w379) -> ("STS"=w376:dbl)  [unwired: 9 in]
            n173 = local write "Sat Id-Log-Used"(w380) -> ()
            n174 = local read "Re-Calculated Values Cluster"() -> (w378:T9)
            n175 = Bundle By Name(cluster=w378, "STS"=w376) -> (w377:T9)
            n176 = local write "Re-Calculated Values Cluster"(w377) -> ()
            n177 = Build Array (concatenate)(w374, w375, w365) -> (w373:cluster{dbl[], dbl[]}[])
            n178 = local write "Sat-Log"(w373) -> ()
          }
          event "Lin-Log Slider": Value Change {
            # "No Indicator for Lin-Log Slider Use"
            n179 = event-data() -> ()  [unwired: 1 in, 5 out]
            n180 = local read "Log-Lin"() -> (w388:cluster{dbl[], dbl[]}[])
            n181 = Decimate 1D Array(w388) -> (w394:cluster{dbl[], dbl[]}[], w395:cluster{dbl[], dbl[]}[])
            n182 = local read "Slider Min"() -> (w391:dbl)
            n183 = Array To Cluster(array=w394) -> (cluster=w401:T16)
            n184 = local read "Num Pts Log"() -> (w398:dbl)
            n185 = local read "Lin-Log Slider"() -> (w389:dbl)
            n186 = Unbundle(w401) -> ("[0]"=w400:cluster{dbl[], dbl[]})  [unwired: 8 out]
            n187 = Absolute Value(x=w391) -> (abs(x)=w390:dbl)
            n188 = Unbundle(w400) -> (w392:dbl[], w399:dbl[])
            n189 = Add(x=w389, y=w390) -> (x+y=w387:dbl)
            n190 = Array Subset(array=w392, index=w387, length=w398) -> (w396:dbl[])
            n191 = local write "Lin-Vg Array-Log Used"(w396) -> ()
            n192 = Array Subset(array=w399, index=w387, length=w398) -> (w397:dbl[])
            n193 = local write "IndexLog-Sat"(w387) -> ()
            n194 = Bundle(w396, w397) -> (w386:cluster{dbl[], dbl[]})  [unwired: 1 in]
            n195 = call "STS-Used.vi"("Id Used"=w397, "Vg-Used"=w396) -> ()  [unwired: 9 in, 1 out]
            n196 = local write "Lin Id-Log Used"(w397) -> ()
            n197 = Build Array (concatenate)(w394, w395, w386) -> (w393:cluster{dbl[], dbl[]}[])
            n198 = local write "Log-Lin"(w393) -> ()
          }
        }
        n199 = Bundle(w66, w63, w66, w66) -> ()  [unwired: 1 in, 1 out]
      }
      frame "Read Data" {
        n200 = call "Recorded Values.vi"("Path"=w445) -> ("Recorded Char"=w463:T9, "Recorded Prop"=w453:T1, "Fabrication Prop"=w447:T4)  [unwired: 8 in]
        n201 = Strip Path(path=w445) -> (stripped path=w446:path, name=w444:string)
        n202 = local write "Fabrication Prop"(w447) -> ()
        n203 = local write "Recorded Prop"(w453) -> ()
        n204 = Unbundle By Name(w453) -> ("Date Recorded"=w452:string, "Index"=w450:string, "Length"=w451:dbl, "Width"=w449:dbl, "Sample Temp"=w448:dbl)
        n205 = local write "Recorded Values Cluster"(w463) -> ()
        n206 = Unbundle By Name(w453) -> ("Sample Temp"=w456:dbl)
        n207 = Unbundle By Name(w447) -> ("Dielectric (nm)"=w441:dbl, "Comments"=w440:string)
        n208 = List Folder(path=w446) -> (filenames=w442:string[])  [unwired: 3 in, 3 out]
        n209 = local write "Rec: Dielectric (d)"(w441) -> ()
        n210 = local write "Date Created"(w452) -> ()
        n211 = local write "Index"(w450) -> ()
        n212 = local write "Rec: Length"(w451) -> ()
        n213 = local write "Rec: Width"(w449) -> ()
        n214 = local write "Rec: Temp"(w448) -> ()
        n215 = Equal To 0?(x=w456) -> (x = 0?=w459:bool)
        n216 = Number To Decimal String(number=w456) -> (decimal integer string=w460:string)  [unwired: 1 in]
        n217 = local write "Comments:"(w440) -> ()
        n218 = Search 1D Array(1D array=w442, element=w444) -> (index of element=w439:i32)  [unwired: 1 in]
        n219 = Equal?(x="", y=w460) -> (x = y?=w458:bool)
        n220 = Index Array(array=w442, index=w439) -> (element=w443:string)
        n221 = Or(x=w459, y=w458) -> (x .or. y?=w457:bool)
        n222 = local write "Data Name:"(w443) -> ()
        n223 = case shown="False" w457 {
          tunnel: [w464 w465] -> w454
          tunnel: w456 -> [w464 _]
          frame False {
          }
          frame True {
            n224 = local read "Room Temp"() -> (w465:dbl)
          }
        }
        n225 = local write "New: Temp"(w454) -> ()
        n226 = Bundle By Name(cluster=w453, "Sample Temp"=w454) -> (w455:T1)
        n227 = local write "Recorded Prop"(w455) -> ()
      }
      frame "Calculated Values" {
        n228 = case shown="True" w466 {
          tunnel: w480 -> [_ w523]
          frame False {
          }
          frame True {
            n229 = local read "Transport Style Controls"() -> (w522:T10)
            n230 = call "TRF to TSP Plot.vi"("Transport Graph Properties"=w522, "Transfer File"=w523) -> ("Transport"=w521:cluster{ext[], ext[]}[])  [unwired: 7 in, 2 out]
            n231 = Array Size(array=w521) -> (size(s)=w520:i32)
            n232 = local write "Transport"(w521) -> ()
            n233 = for {
              N: w520 -> [_]
              tunnel: w522 -> [w527]
              i -> [w526]
              n234 = Unbundle By Name(w527) -> ("Transport Line Size"=w524:u16, "Transport Line Color"=w525:u32)
              n235 = property on="Transport" class="XYGraph (strict)"("Active Plot"=w526, "Plot.Plot Color"=w525, "Plot.Line Width"=w524) -> ()  [unwired: 2 in, 2 out]
            }
          }
        }
        n236 = local read "Fabrication Prop"() -> (w509:T4)
        n237 = local read "Recorded Prop"() -> (w502:T1)
        n238 = local read "Calculated Values Cluster"() -> (w519:T9)
        n239 = call "Mobility-Vt Calculator-File.vi"("NumPts"=w504, "Path"=w480) -> ("Used Points"=w497:T17, "Graph Cluster"=w486:T18, "Lin Vd"=w493:dbl, "Output"=w517:T19)  [unwired: 6 in]
        n240 = call "STS Calculator-File.vi"("NumPts"=w503, "Path"=w480) -> ("Used Points"=w491:T20, "XY Graph-Sat"=w473:cluster{dbl[], dbl[]}[], "XY Graph-Lin"=w474:cluster{dbl[], dbl[]}[], "Ouput"=w512:cluster{"STS-Sat":dbl, "STS-Lin":dbl})  [unwired: 6 in]
        n241 = Unbundle By Name(w509) -> ("Dielectric (nm)"=w507:dbl)
        n242 = Unbundle By Name(w502) -> ("Sample Temp"=w501:dbl)
        n243 = Unbundle By Name(w517) -> ("Mobility-Sat"=w516:dbl, "Vt-Sat"=w508:dbl, "Mobility-Lin"=w515:dbl, "Off I-Sat"=w514:dbl, "On/Off I-Sat"=w513:dbl)  [unwired: 1 out]
        n244 = local write "Lin Vd"(w493) -> ()
        n245 = Unbundle By Name(w512) -> ("STS-Sat"=w506:dbl)  [unwired: 1 out]
        n246 = local write "Sat-Log"(w473) -> ()
        n247 = local write "Log-Lin"(w474) -> ()
        n248 = call "Trap Density_VT.vi"("VT"=w508, "Dielectric"=w507) -> ("Trap Density-VT"=w511:dbl)
        n249 = call "Trap Density_STS.vi"("Temp (T) [K]"=w501, "S.T.S. (S)"=w506, "Dielectric"=w507) -> ("Trap Density (N)"=w510:dbl)  [unwired: 8 in]
        n250 = call "Image from TRF Display.vi"("No Image File"=w499, "Image Folder"=w500, "Transfer File"=w480) -> ("Image Out 2"=w467:T8, "Image Out"=w468:T8, "Image File"=w469:path, "Image Name"=w470:string)  [unwired: 5 in]
        n251 = Bundle By Name(cluster=w519, "Mobility-Sat"=w516, "Moblitity-Lin"=w515, "On/Off"=w513, "Off Current"=w514, "Vt-Sat"=w508, "STS"=w506, "Trap Density-VT"=w511, "Trap Density-STS"=w510) -> (w518:T9)
        n252 = Unbundle By Name(w491) -> ("Sat Vg Used"=w490:dbl[], "Sat Log(Id) Used"=w489:dbl[], "Lin Vg Used"=w488:dbl[], "Lin Log(Id) Used"=w487:dbl[], "STS Index-Sat"=w471:dbl, "STS Index-Lin"=w472:dbl)
        n253 = Unbundle By Name(w497) -> ("Sat Vg Used"=w496:dbl[], "Sat Sqrt(Id) Used"=w495:dbl[], "Lin Vg Used"=w494:dbl[], "Lin Sqrt(Id) Used"=w492:dbl[], "Index-Lin"=w482:dbl, "Index-Sat"=w481:dbl)
        n254 = local write "Image File"(w469) -> ()
        n255 = local write "Image Name"(w470) -> ()
        n256 = local write "Image Out"(w468) -> ()
        n257 = local write "Image Preview"(w467) -> ()
        n258 = local write "Vg Array-Log-Used"(w490) -> ()
        n259 = local write "Sat Id-Log-Used"(w489) -> ()
        n260 = local write "Lin-Vg Array-Log Used"(w488) -> ()
        n261 = local write "Lin Id-Log Used"(w487) -> ()
        n262 = local write "IndexLog-Sat"(w471) -> ()
        n263 = local write "Index-Lin"(w472) -> ()
        n264 = local write "Calculated Values Cluster"(w518) -> ()
        n265 = local write "Sat Vg Array-Used"(w496) -> ()
        n266 = local write "Sat Id-Used"(w495) -> ()
        n267 = local write "Lin-Vg Array-Used"(w494) -> ()
        n268 = local write "Lin Id-Used"(w492) -> ()
        n269 = local write "Index-Sat"(w481) -> ()
        n270 = local write "Index-Lin"(w482) -> ()
        n271 = local write "Lin-Log Slider"(w472) -> ()
        n272 = local write "Sat-Log Slider"(w471) -> ()
        n273 = local write "Sat-Trans Slider"(w481) -> ()
        n274 = local write "Lin-Trans Slider"(w482) -> ()
        n275 = Unbundle By Name(w486) -> ("Raw Sat"=w479:cluster{dbl[], dbl[]}[], "Sqrt Sat"=w483:cluster{dbl[], dbl[]}[], "Raw Lin"=w485:cluster{dbl[], dbl[]}[], "Sqrt Lin"=w484:cluster{dbl[], dbl[]}[])
        n276 = Index Array(array=w479) -> (element=w478:cluster{dbl[], dbl[]})  [unwired: 1 in]
        n277 = Unbundle(w478) -> (w477:dbl[])  [unwired: 1 out]
        n278 = Array Max & Min(array=w477) -> (max value=w476:dbl, min value=w475:dbl)  [unwired: 2 out]
        n279 = property on="Sat-Trans Slider" class="Slide (strict)"("Scale.Maximum"=w476, "Scale.Minimum"=w475) -> ()  [unwired: 2 in, 2 out]
        n280 = property on="Lin-Trans Slider" class="Slide (strict)"("Scale.Maximum"=w476, "Scale.Minimum"=w475) -> ()  [unwired: 2 in, 2 out]
        n281 = property on="Sat-Log Slider" class="Slide (strict)"("Scale.Maximum"=w476, "Scale.Minimum"=w475) -> ()  [unwired: 2 in, 2 out]
        n282 = property on="Lin-Log Slider" class="Slide (strict)"("Scale.Maximum"=w476, "Scale.Minimum"=w475) -> ()  [unwired: 2 in, 2 out]
        n283 = local write "Slider Max"(w476) -> ()
        n284 = local write "Slider Min"(w475) -> ()
        n285 = local write "Raw- Sat"(w479) -> ()
        n286 = local write "Raw- Lin"(w485) -> ()
        n287 = local write "Sqrt-Sat"(w483) -> ()
        n288 = local write "Sqrt-Lin"(w484) -> ()
      }
      frame "Re-Calculated Values" {
        n289 = local read "Vg Array-Log-Used"() -> (w536:dbl[])
        n290 = local read "Sat Vg Array-Used"() -> (w544:dbl[])
        n291 = local read "Lin-Vg Array-Used"() -> (w550:dbl[])
        n292 = local read "Sat Id-Log-Used"() -> (w535:dbl[])
        n293 = local read "New: Dielectric"() -> (w548:dbl)
        n294 = local read "New: Dielectric"() -> (w533:dbl)
        n295 = local read "New: Length"() -> (w547:dbl)
        n296 = local read "New: Length"() -> (w543:dbl)
        n297 = local read "New: Width"() -> (w546:dbl)
        n298 = local read "New: Width"() -> (w542:dbl)
        n299 = local read "Lin Id-Used"() -> (w549:dbl[])
        n300 = local read "Sat Id-Used"() -> (w541:dbl[])
        n301 = local read "Re-Calculated Values Cluster"() -> (w552:T9)
        n302 = local read "New: Dielectric"() -> (w532:dbl)
        n303 = local read "New: Temp"() -> (w531:dbl)
        n304 = local read "Lin Vd"() -> (w528:dbl)
        n305 = call "Mobility-Vt-Used Pts_Saturation.vi"("Width"=w542, "Length"=w543, "Dielectric (d)"=w533, "Sat Id Used"=w541, "Vg Used"=w544) -> ("Vt"=w539:dbl, "Mobility"=w540:dbl)  [unwired: 4 in, 1 out]
        n306 = call "STS-Used.vi"("Id Used"=w535, "Vg-Used"=w536) -> ("STS"=w534:dbl)  [unwired: 9 in]
        n307 = call "Mobility-Vt-Used Pts_Linear.vi"("Width"=w546, "Length"=w547, "Vd"=w528, "Dielectric (d)"=w548, "Id Used"=w549, "Vg Used"=w550) -> ("Mobility"=w545:dbl)  [unwired: 3 in, 2 out]
        n308 = call "Trap Density_VT.vi"("VT"=w539, "Dielectric"=w533) -> ("Trap Density-VT"=w538:dbl)
        n309 = call "Trap Density_STS.vi"("Temp (T) [K]"=w531, "S.T.S. (S)"=w534, "Dielectric"=w532) -> ("Trap Density (N)"=w530:dbl)  [unwired: 8 in]
        n310 = Bundle By Name(cluster=w552, "Mobility-Sat"=w540, "Moblitity-Lin"=w545, "Vt-Sat"=w539, "STS"=w534, "Trap Density-VT"=w538, "Trap Density-STS"=w530) -> (w551:T9)
        n311 = local write "Re-Calculated Values Cluster"(w551) -> ()
      }
      frame "Next File" {
        n312 = Strip Path(path=w569) -> (stripped path=w559:path, name=w567:string)
        n313 = local write "Transfer Folder"(w559) -> ()
        n314 = List Folder(path=w559) -> (filenames=w553:string[], error out=w562:errorcluster)  [unwired: 3 in, 2 out]
        n315 = Array Size(array=w553) -> (size(s)=w566:i32)
        n316 = Search 1D Array(1D array=w553, element=w567) -> (index of element=w564:i32)  [unwired: 1 in]
        n317 = Decrement(x=w566) -> (x-1=w565:i32)
        n318 = Equal?(x=w565, y=w564) -> (x = y?=w563:bool)
        n319 = case shown="False" w563 {
          tunnel: w555 -> [w572 _]
          tunnel: [w571 0] -> w554
          tunnel: w562 -> [w570 w573]
          tunnel: [w570 w573] -> _
          frame False {
            n320 = Increment(x=w572) -> (x+1=w571:i32)
          }
          frame True {
          }
        }
        n321 = Path To String(path=w559) -> (string=w560:string)
        n322 = Index Array(array=w553, index=w554) -> (element=w561:string)
        n323 = Concatenate Strings(w560, "\\", w561) -> (w557:string)
        n324 = String To Path(string=w557) -> (path=w556:path)
        n325 = local write "Transfer File"(w556) -> ()
      }
      frame "Previous File" {
        n326 = Strip Path(path=w581) -> (stripped path=w578:path, name=w590:string)
        n327 = local write "Transfer Folder"(w578) -> ()
        n328 = List Folder(path=w578) -> (filenames=w582:string[], error out=w587:errorcluster)  [unwired: 3 in, 2 out]
        n329 = Array Size(array=w582) -> (size(s)=w576:i32)
        n330 = Search 1D Array(1D array=w582, element=w590) -> (index of element=w589:i32)  [unwired: 1 in]
        n331 = Decrement(x=w576) -> (x-1=w575:i32)
        n332 = Equal To 0?(x=w589) -> (x = 0?=w588:bool)
        n333 = case shown="False" w588 {
          tunnel: w580 -> [w594 _]
          tunnel: [w593 w595] -> w579
          tunnel: w587 -> [w592 w596]
          tunnel: [w592 w596] -> _
          tunnel: w575 -> [_ w595]
          frame False {
            n334 = Decrement(x=w594) -> (x-1=w593:i32)
          }
          frame True {
          }
        }
        n335 = Path To String(path=w578) -> (string=w577:string)
        n336 = Index Array(array=w582, index=w579) -> (element=w586:string)
        n337 = Concatenate Strings(w577, "\\", w586) -> (w584:string)
        n338 = String To Path(string=w584) -> (path=w583:path)
        n339 = local write "Transfer File"(w583) -> ()
      }
      frame "Discard File" {
      }
      frame "Save" {
        n340 = stacked-sequence {
          seq-local: [w614 _] -> [_ w1111]
          seq-local: [w613 _] -> [_ w1109]
          tunnel: w605 -> [w615 w1112]
          frame #0 {
            # "Saves each Re-calculated parameter in sequence"
            n341 = stacked-sequence {
              tunnel: [_ _ _ _ _ _ _ _ _ _ _ _ _ w1079] -> w613
              tunnel: w615 -> [w635 _ _ _ _ _ _ _ _ _ _ _ _ _]
              frame #0 {
                n342 = call-poly <vilib>:"Read From Spreadsheet File.vi"("file path (dialog if empty)"=w635) -> ("all rows"=w634:string[][])  [unwired: 6 in, 4 out]
                n343 = Array Size(array=w634) -> (size(s)=w639:i32[])
                n344 = Array Subset(array=w634, index (row)=0, index (col)=0, length (col)=3) -> (w643:string[][])  [unwired: 1 in]
                n345 = Index Array(array=w639, index=0) -> (element=w637:i32)
                n346 = Reshape Array(w643, w637) -> (w636:string[])
                n347 = Search 1D Array(1D array=w636, element="Dielectric (nm):") -> (index of element=w646:i32)  [unwired: 1 in]
                n348 = Equal?(x=w646, y=-1) -> (x = y?=w645:bool)
                n349 = case shown="False" w645 {
                  tunnel: w634 -> [w654 w658]
                  tunnel: w646 -> [w650 _]
                  tunnel: [w649 w658] -> w644
                  frame False {
                    n350 = local read "Rec: Dielectric (d)"() -> (w656:dbl)
                    n351 = Number To Fractional String(number=w656) -> (F-format string=w651:string)  [unwired: 3 in]
                    n352 = Divide(x=w650, y=3) -> (x/y=w653:dbl)
                    n353 = To Word Integer(number=w653) -> (16bit integer=w652:i16)
                    n354 = Replace Array Subset(array=w654, new element=w651, index (row)=w652, index (col)=1) -> (w649:string[][])
                  }
                  frame True {
                  }
                }
                n355 = local write "Save Array"(w644) -> ()
              }
              frame #1 {
                n356 = local read "Save Array"() -> (w660:string[][])
                n357 = Array Size(array=w660) -> (size(s)=w663:i32[])
                n358 = Array Subset(array=w660, index (row)=0, index (col)=0, length (col)=3) -> (w667:string[][])  [unwired: 1 in]
                n359 = Index Array(array=w663, index=0) -> (element=w661:i32)
                n360 = Reshape Array(w667, w661) -> (w659:string[])
                n361 = Search 1D Array(1D array=w659, element="Comments:") -> (index of element=w670:i32)  [unwired: 1 in]
                n362 = Equal?(x=w670, y=-1) -> (x = y?=w669:bool)
                n363 = case shown="False" w669 {
                  tunnel: w660 -> [w678 w681]
                  tunnel: w670 -> [w675 _]
                  tunnel: [w674 w681] -> w668
                  frame False {
                    n364 = local read "New: Comments"() -> (w673:string)
                    n365 = Divide(x=w675, y=3) -> (x/y=w677:dbl)
                    n366 = To Word Integer(number=w677) -> (16bit integer=w676:i16)
                    n367 = Replace Array Subset(array=w678, new element=w673, index (row)=w676, index (col)=1) -> (w674:string[][])
                  }
                  frame True {
                  }
                }
                n368 = local write "Save Array"(w668) -> ()
              }
              frame #2 {
                n369 = local read "Save Array"() -> (w683:string[][])
                n370 = Array Size(array=w683) -> (size(s)=w686:i32[])
                n371 = Array Subset(array=w683, index (row)=0, index (col)=0, length (col)=3) -> (w690:string[][])  [unwired: 1 in]
                n372 = Index Array(array=w686, index=0) -> (element=w684:i32)
                n373 = Reshape Array(w690, w684) -> (w682:string[])
                n374 = Search 1D Array(1D array=w682, element="Length (um):") -> (index of element=w693:i32)  [unwired: 1 in]
                n375 = Equal?(x=w693, y=-1) -> (x = y?=w692:bool)
                n376 = case shown="False" w692 {
                  tunnel: w683 -> [w703 w706]
                  tunnel: w693 -> [w700 _]
                  tunnel: [w699 w706] -> w691
                  frame False {
                    n377 = local read "New: Length"() -> (w696:dbl)
                    n378 = Divide(x=w700, y=3) -> (x/y=w702:dbl)
                    n379 = Format Value(format string="%#g", value (0)=w696) -> (output string=w697:string)  [unwired: 1 in]
                    n380 = To Word Integer(number=w702) -> (16bit integer=w701:i16)
                    n381 = Replace Array Subset(array=w703, new element=w697, index (row)=w701, index (col)=1) -> (w699:string[][])
                  }
                  frame True {
                  }
                }
                n382 = local write "Save Array"(w691) -> ()
              }
              frame #3 {
                n383 = local read "Save Array"() -> (w708:string[][])
                n384 = Array Size(array=w708) -> (size(s)=w713:i32[])
                n385 = Array Subset(array=w708, index (row)=0, index (col)=0, length (col)=3) -> (w709:string[][])  [unwired: 1 in]
                n386 = Index Array(array=w713, index=0) -> (element=w715:i32)
                n387 = Reshape Array(w709, w715) -> (w707:string[])
                n388 = Search 1D Array(1D array=w707, element="Width (um):") -> (index of element=w718:i32)  [unwired: 1 in]
                n389 = Equal?(x=w718, y=-1) -> (x = y?=w717:bool)
                n390 = case shown="False" w717 {
                  tunnel: w718 -> [w726 _]
                  tunnel: w708 -> [w725 w731]
                  tunnel: [w724 w731] -> w716
                  frame False {
                    n391 = local read "New: Width"() -> (w721:dbl)
                    n392 = Divide(x=w726, y=3) -> (x/y=w728:dbl)
                    n393 = To Word Integer(number=w728) -> (16bit integer=w727:i16)
                    n394 = Format Value(format string="%#g", value (0)=w721) -> (output string=w722:string)  [unwired: 1 in]
                    n395 = Replace Array Subset(array=w725, new element=w722, index (row)=w727, index (col)=1) -> (w724:string[][])
                  }
                  frame True {
                  }
                }
                n396 = local write "Save Array"(w716) -> ()
              }
              frame #4 {
                w741 = "Sample Temp (K):"
                n397 = local read "Save Array"() -> (w733:string[][])
                n398 = Array Size(array=w733) -> (size(s)=w738:i32[])
                n399 = Array Subset(array=w733, index (row)=0, index (col)=0, length (col)=3) -> (w734:string[][])  [unwired: 1 in]
                n400 = Index Array(array=w738, index=0) -> (element=w740:i32)
                n401 = Reshape Array(w734, w740) -> (w732:string[])
                n402 = Search 1D Array(1D array=w732, element=w741) -> (index of element=w744:i32)  [unwired: 1 in]
                n403 = Equal?(x=w744, y=-1) -> (x = y?=w743:bool)
                n404 = case shown="False" w743 {
                  tunnel: w733 -> [w753 w767]
                  tunnel: w744 -> [w750 _]
                  tunnel: [w749 w766] -> w742
                  tunnel: w732 -> [_ w769]
                  tunnel: w741 -> [_ w756]
                  frame False {
                    n405 = local read "New: Temp"() -> (w747:dbl)
                    n406 = Divide(x=w750, y=3) -> (x/y=w752:dbl)
                    n407 = Format Value(format string="%#g", value (0)=w747) -> (output string=w746:string)  [unwired: 1 in]
                    n408 = To Word Integer(number=w752) -> (16bit integer=w751:i16)
                    n409 = Replace Array Subset(array=w753, new element=w746, index (row)=w751, index (col)=1) -> (w749:string[][])
                  }
                  frame True {
                    n410 = local read "New: Temp"() -> (w758:dbl)
                    n411 = Search 1D Array(1D array=w769, element="Width (um):") -> (index of element=w763:i32)  [unwired: 1 in]
                    n412 = Divide(x=w763, y=3) -> (x/y=w764:dbl)
                    n413 = To Word Integer(number=w764) -> (16bit integer=w762:i16)
                    n414 = Format Value(format string="%#g", value (0)=w758) -> (output string=w757:string)  [unwired: 1 in]
                    n415 = Build Array(w756, w757) -> (w760:string[])
                    n416 = Increment(x=w762) -> (x+1=w761:i16)
                    n417 = Insert Into Array(array=w767, index (row)=w761, new element=w760) -> (w766:string[][])  [unwired: 1 in]
                  }
                }
                n418 = local write "Save Array"(w742) -> ()
              }
              frame #5 {
                w779 = "Mobility-Sat (cm^2/Vs):"
                n419 = local read "Save Array"() -> (w771:string[][])
                n420 = Array Size(array=w771) -> (size(s)=w776:i32[])
                n421 = Array Subset(array=w771, index (row)=0, index (col)=0, length (col)=3) -> (w772:string[][])  [unwired: 1 in]
                n422 = Index Array(array=w776, index=0) -> (element=w778:i32)
                n423 = Reshape Array(w772, w778) -> (w770:string[])
                n424 = Search 1D Array(1D array=w770, element=w779) -> (index of element=w782:i32)  [unwired: 1 in]
                n425 = Equal?(x=w782, y=-1) -> (x = y?=w781:bool)
                n426 = case shown="False" w781 {
                  tunnel: w771 -> [w792 w802]
                  tunnel: w782 -> [w789 _]
                  tunnel: [w788 w801] -> w780
                  tunnel: w770 -> [_ w799]
                  tunnel: w779 -> [_ w797]
                  frame False {
                    n427 = local read "Re-Calculated Values Cluster"() -> (w785:T9)
                    n428 = Unbundle By Name(w785) -> ("Mobility-Sat"=w784:dbl)
                    n429 = Divide(x=w789, y=3) -> (x/y=w791:dbl)
                    n430 = To Word Integer(number=w791) -> (16bit integer=w790:i16)
                    n431 = Format Value(format string="%#g", value (0)=w784) -> (output string=w786:string)  [unwired: 1 in]
                    n432 = Replace Array Subset(array=w792, new element=w786, index (row)=w790, index (col)=1) -> (w788:string[][])
                  }
                  frame True {
                    n433 = local read "Re-Calculated Values Cluster"() -> (w796:T9)
                    n434 = Unbundle By Name(w796) -> ("Mobility-Sat"=w795:dbl)
                    n435 = Search 1D Array(1D array=w799, element="Mobility (cm^2/Vs):") -> (index of element=w805:i32)  [unwired: 1 in]
                    n436 = Divide(x=w805, y=3) -> (x/y=w806:dbl)
                    n437 = To Word Integer(number=w806) -> (16bit integer=w798:i16)
                    n438 = Format Value(format string="%#g", value (0)=w795) -> (output string=w800:string)  [unwired: 1 in]
                    n439 = Build Array(w797, w800) -> (w804:string[])
                    n440 = Replace Array Subset(array=w802, new element=w804, index (row)=w798) -> (w801:string[][])  [unwired: 1 in]
                  }
                }
                n441 = local write "Save Array"(w780) -> ()
              }
              frame #6 {
                w818 = "Mobility-Lin (cm^2/Vs):"
                n442 = local read "Save Array"() -> (w809:string[][])
                n443 = Array Size(array=w809) -> (size(s)=w815:i32[])
                n444 = Array Subset(array=w809, index (row)=0, index (col)=0, length (col)=3) -> (w811:string[][])  [unwired: 1 in]
                n445 = Index Array(array=w815, index=0) -> (element=w817:i32)
                n446 = Reshape Array(w811, w817) -> (w810:string[])
                n447 = Search 1D Array(1D array=w810, element=w818) -> (index of element=w821:i32)  [unwired: 1 in]
                n448 = Equal?(x=w821, y=-1) -> (x = y?=w820:bool)
                n449 = case shown="True" w820 {
                  tunnel: w809 -> [w831 w839]
                  tunnel: w821 -> [w828 _]
                  tunnel: [w827 w838] -> w819
                  tunnel: w810 -> [_ w837]
                  tunnel: w818 -> [_ w836]
                  frame False {
                    n450 = local read "Re-Calculated Values Cluster"() -> (w824:T9)
                    n451 = Unbundle By Name(w824) -> ("Moblitity-Lin"=w823:dbl)
                    n452 = Divide(x=w828, y=3) -> (x/y=w830:dbl)
                    n453 = To Word Integer(number=w830) -> (16bit integer=w829:i16)
                    n454 = Format Value(format string="%#g", value (0)=w823) -> (output string=w825:string)  [unwired: 1 in]
                    n455 = Replace Array Subset(array=w831, new element=w825, index (row)=w829, index (col)=1) -> (w827:string[][])
                  }
                  frame True {
                    n456 = local read "Re-Calculated Values Cluster"() -> (w835:T9)
                    n457 = Unbundle By Name(w835) -> ("Moblitity-Lin"=w834:dbl)
                    n458 = Search 1D Array(1D array=w837, element="Mobility-Sat (cm^2/Vs):") -> (index of element=w844:i32)  [unwired: 1 in]
                    n459 = Divide(x=w844, y=3) -> (x/y=w845:dbl)
                    n460 = To Word Integer(number=w845) -> (16bit integer=w843:i16)
                    n461 = Format Value(format string="%#g", value (0)=w834) -> (output string=w848:string)  [unwired: 1 in]
                    n462 = Build Array(w836, w848) -> (w841:string[])
                    n463 = Increment(x=w843) -> (x+1=w842:i16)
                    n464 = Insert Into Array(array=w839, index (row)=w842, new element=w841) -> (w838:string[][])  [unwired: 1 in]
                  }
                }
                n465 = local write "Save Array"(w819) -> ()
              }
              frame #7 {
                w858 = "On/Off I-Sat:"
                n466 = local read "Save Array"() -> (w849:string[][])
                n467 = Array Size(array=w849) -> (size(s)=w855:i32[])
                n468 = Array Subset(array=w849, index (row)=0, index (col)=0, length (col)=3) -> (w851:string[][])  [unwired: 1 in]
                n469 = Index Array(array=w855, index=0) -> (element=w857:i32)
                n470 = Reshape Array(w851, w857) -> (w850:string[])
                n471 = Search 1D Array(1D array=w850, element=w858) -> (index of element=w861:i32)  [unwired: 1 in]
                n472 = Equal?(x=w861, y=-1) -> (x = y?=w860:bool)
                n473 = case shown="True" w860 {
                  tunnel: w849 -> [w871 w880]
                  tunnel: w861 -> [w868 _]
                  tunnel: [w867 w881] -> w859
                  tunnel: w850 -> [_ w878]
                  tunnel: w858 -> [_ w876]
                  frame False {
                    n474 = local read "Re-Calculated Values Cluster"() -> (w864:T9)
                    n475 = Divide(x=w868, y=3) -> (x/y=w870:dbl)
                    n476 = Unbundle By Name(w864) -> ("On/Off"=w863:dbl)
                    n477 = To Word Integer(number=w870) -> (16bit integer=w869:i16)
                    n478 = Format Value(format string="%#g", value (0)=w863) -> (output string=w865:string)  [unwired: 1 in]
                    n479 = Replace Array Subset(array=w871, new element=w865, index (row)=w869, index (col)=1) -> (w867:string[][])
                  }
                  frame True {
                    n480 = local read "Re-Calculated Values Cluster"() -> (w875:T9)
                    n481 = Unbundle By Name(w875) -> ("On/Off"=w874:dbl)
                    n482 = Search 1D Array(1D array=w878, element="On/Off Current:") -> (index of element=w884:i32)  [unwired: 1 in]
                    n483 = Divide(x=w884, y=3) -> (x/y=w885:dbl)
                    n484 = To Word Integer(number=w885) -> (16bit integer=w877:i16)
                    n485 = Format Value(format string="%#g", value (0)=w874) -> (output string=w879:string)  [unwired: 1 in]
                    n486 = Build Array(w876, w879) -> (w883:string[])
                    n487 = Replace Array Subset(array=w880, new element=w883, index (row)=w877) -> (w881:string[][])  [unwired: 1 in]
                  }
                }
                n488 = local write "Save Array"(w859) -> ()
              }
              frame #8 {
                w897 = "Off I-Sat (A):"
                n489 = local read "Save Array"() -> (w888:string[][])
                n490 = Array Size(array=w888) -> (size(s)=w894:i32[])
                n491 = Array Subset(array=w888, index (row)=0, index (col)=0, length (col)=3) -> (w890:string[][])  [unwired: 1 in]
                n492 = Index Array(array=w894, index=0) -> (element=w896:i32)
                n493 = Reshape Array(w890, w896) -> (w889:string[])
                n494 = Search 1D Array(1D array=w889, element=w897) -> (index of element=w900:i32)  [unwired: 1 in]
                n495 = Equal?(x=w900, y=-1) -> (x = y?=w899:bool)
                n496 = case shown="True" w899 {
                  tunnel: w888 -> [w910 w918]
                  tunnel: w900 -> [w907 _]
                  tunnel: [w906 w917] -> w898
                  tunnel: w889 -> [_ w916]
                  tunnel: w897 -> [_ w915]
                  frame False {
                    n497 = local read "Re-Calculated Values Cluster"() -> (w903:T9)
                    n498 = Unbundle By Name(w903) -> ("Off Current"=w902:dbl)
                    n499 = Divide(x=w907, y=3) -> (x/y=w909:dbl)
                    n500 = Format Value(format string="%#g", value (0)=w902) -> (output string=w904:string)  [unwired: 1 in]
                    n501 = To Word Integer(number=w909) -> (16bit integer=w908:i16)
                    n502 = Replace Array Subset(array=w910, new element=w904, index (row)=w908, index (col)=1) -> (w906:string[][])
                  }
                  frame True {
                    n503 = local read "Re-Calculated Values Cluster"() -> (w914:T9)
                    n504 = Unbundle By Name(w914) -> ("Off Current"=w913:dbl)
                    n505 = Search 1D Array(1D array=w916, element="On/Off I-Sat:") -> (index of element=w923:i32)  [unwired: 1 in]
                    n506 = Divide(x=w923, y=3) -> (x/y=w924:dbl)
                    n507 = To Word Integer(number=w924) -> (16bit integer=w922:i16)
                    n508 = Format Value(format string="%#g", value (0)=w913) -> (output string=w927:string)  [unwired: 1 in]
                    n509 = Build Array(w915, w927) -> (w920:string[])
                    n510 = Increment(x=w922) -> (x+1=w921:i16)
                    n511 = Insert Into Array(array=w918, index (row)=w921, new element=w920) -> (w917:string[][])  [unwired: 1 in]
                  }
                }
                n512 = local write "Save Array"(w898) -> ()
              }
              frame #9 {
                w929 = "Vt-Sat (V):"
                n513 = local read "Save Array"() -> (w930:string[][])
                n514 = Array Size(array=w930) -> (size(s)=w935:i32[])
                n515 = Array Subset(array=w930, index (row)=0, index (col)=0, length (col)=3) -> (w931:string[][])  [unwired: 1 in]
                n516 = Index Array(array=w935, index=0) -> (element=w937:i32)
                n517 = Reshape Array(w931, w937) -> (w928:string[])
                n518 = Search 1D Array(1D array=w928, element=w929) -> (index of element=w940:i32)  [unwired: 1 in]
                n519 = Equal?(x=w940, y=-1) -> (x = y?=w939:bool)
                n520 = case shown="False" w939 {
                  tunnel: w930 -> [w949 w959]
                  tunnel: w940 -> [w945 _]
                  tunnel: [w944 w958] -> w938
                  tunnel: w929 -> [_ w957]
                  tunnel: w928 -> [_ w956]
                  frame False {
                    n521 = local read "Re-Calculated Values Cluster"() -> (w943:T9)
                    n522 = Unbundle By Name(w943) -> ("Vt-Sat"=w942:dbl)
                    n523 = Divide(x=w945, y=3) -> (x/y=w948:dbl)
                    n524 = To Word Integer(number=w948) -> (16bit integer=w947:i16)
                    n525 = Number To Fractional String(number=w942) -> (F-format string=w946:string)  [unwired: 3 in]
                    n526 = Replace Array Subset(array=w949, new element=w946, index (row)=w947, index (col)=1) -> (w944:string[][])
                  }
                  frame True {
                    n527 = local read "Re-Calculated Values Cluster"() -> (w953:T9)
                    n528 = Unbundle By Name(w953) -> ("Vt-Sat"=w952:dbl)
                    n529 = Search 1D Array(1D array=w956, element="Threshold V (V):") -> (index of element=w955:i32)  [unwired: 1 in]
                    n530 = Divide(x=w955, y=3) -> (x/y=w962:dbl)
                    n531 = To Word Integer(number=w962) -> (16bit integer=w954:i16)
                    n532 = Format Value(format string="%#g", value (0)=w952) -> (output string=w965:string)  [unwired: 1 in]
                    n533 = Build Array(w957, w965) -> (w961:string[])
                    n534 = Replace Array Subset(array=w959, new element=w961, index (row)=w954) -> (w958:string[][])  [unwired: 1 in]
                  }
                }
                n535 = local write "Save Array"(w938) -> ()
              }
              frame #10 {
                n536 = disable-structure shown="Disabled" {
                  frame Disabled {
                    n537 = local read "Save Array"() -> (w966:string[][])
                    n538 = Array Size(array=w966) -> (size(s)=w972:i32[])
                    n539 = Array Subset(array=w966, index (row)=0, index (col)=0, length (col)=3) -> (w968:string[][])  [unwired: 1 in]
                    n540 = Index Array(array=w972, index=0) -> (element=w974:i32)
                    n541 = Reshape Array(w968, w974) -> (w967:string[])
                    n542 = Search 1D Array(1D array=w967, element="VT-Lin (V):") -> (index of element=w977:i32)  [unwired: 1 in]
                    n543 = Equal?(x=w977, y=-1) -> (x = y?=w976:bool)
                    n544 = case shown="False" w976 {
                      tunnel: w966 -> [w986 w989]
                      tunnel: w977 -> [w983 _]
                      tunnel: [w982 w989] -> w975
                      frame False {
                        n545 = Divide(x=w983, y=3) -> (x/y=w985:dbl)
                        n546 = To Word Integer(number=w985) -> (16bit integer=w984:i16)
                        n547 = Format Value(format string="%#g") -> (output string=w980:string)  [unwired: 2 in]
                        n548 = Replace Array Subset(array=w986, new element=w980, index (row)=w984, index (col)=1) -> (w982:string[][])
                      }
                      frame True {
                      }
                    }
                    n549 = local write "Save Array"(w975) -> ()
                  }
                  frame Enabled {
                  }
                }
              }
              frame #11 {
                w990 = "STS-Sat (V/decade):"
                n550 = local read "Save Array"() -> (w992:string[][])
                n551 = Array Size(array=w992) -> (size(s)=w997:i32[])
                n552 = Array Subset(array=w992, index (row)=0, index (col)=0, length (col)=3) -> (w993:string[][])  [unwired: 1 in]
                n553 = Index Array(array=w997, index=0) -> (element=w999:i32)
                n554 = Reshape Array(w993, w999) -> (w991:string[])
                n555 = Search 1D Array(1D array=w991, element=w990) -> (index of element=w1002:i32)  [unwired: 1 in]
                n556 = Equal?(x=w1002, y=-1) -> (x = y?=w1001:bool)
                n557 = case shown="True" w1001 {
                  tunnel: w992 -> [w1012 w1020]
                  tunnel: w1002 -> [w1009 _]
                  tunnel: [w1008 w1021] -> w1000
                  tunnel: w991 -> [_ w1019]
                  tunnel: w990 -> [_ w1018]
                  frame False {
                    n558 = local read "Re-Calculated Values Cluster"() -> (w1004:T9)
                    n559 = Unbundle By Name(w1004) -> ("STS"=w1005:dbl)
                    n560 = Divide(x=w1009, y=3) -> (x/y=w1011:dbl)
                    n561 = To Word Integer(number=w1011) -> (16bit integer=w1010:i16)
                    n562 = Format Value(format string="%#g", value (0)=w1005) -> (output string=w1006:string)  [unwired: 1 in]
                    n563 = Replace Array Subset(array=w1012, new element=w1006, index (row)=w1010, index (col)=1) -> (w1008:string[][])
                  }
                  frame True {
                    n564 = local read "Re-Calculated Values Cluster"() -> (w1015:T9)
                    n565 = Unbundle By Name(w1015) -> ("STS"=w1016:dbl)
                    n566 = Search 1D Array(1D array=w1019, element="S.T.S. (V/decade):") -> (index of element=w1024:i32)  [unwired: 1 in]
                    n567 = Divide(x=w1024, y=3) -> (x/y=w1025:dbl)
                    n568 = To Word Integer(number=w1025) -> (16bit integer=w1017:i16)
                    n569 = Format Value(format string="%#g", value (0)=w1016) -> (output string=w1028:string)  [unwired: 1 in]
                    n570 = Build Array(w1018, w1028) -> (w1023:string[])
                    n571 = Replace Array Subset(array=w1020, new element=w1023, index (row)=w1017) -> (w1021:string[][])  [unwired: 1 in]
                  }
                }
                n572 = local write "Save Array"(w1000) -> ()
              }
              frame #12 {
                w1029 = "Trap Density-VT (Traps/Vcm^2):"
                n573 = local read "Save Array"() -> (w1031:string[][])
                n574 = Array Size(array=w1031) -> (size(s)=w1036:i32[])
                n575 = Array Subset(array=w1031, index (row)=0, index (col)=0, length (col)=3) -> (w1032:string[][])  [unwired: 1 in]
                n576 = Index Array(array=w1036, index=0) -> (element=w1038:i32)
                n577 = Reshape Array(w1032, w1038) -> (w1030:string[])
                n578 = Search 1D Array(1D array=w1030, element=w1029) -> (index of element=w1041:i32)  [unwired: 1 in]
                n579 = Equal?(x=w1041, y=-1) -> (x = y?=w1040:bool)
                n580 = case shown="True" w1040 {
                  tunnel: w1031 -> [w1051 w1058]
                  tunnel: w1041 -> [w1047 _]
                  tunnel: [w1046 w1059] -> w1039
                  tunnel: w1030 -> [_ w1057]
                  tunnel: w1029 -> [_ w1056]
                  frame False {
                    n581 = local read "Re-Calculated Values Cluster"() -> (w1044:T9)
                    n582 = Unbundle By Name(w1044) -> ("Trap Density-VT"=w1043:dbl)
                    n583 = Divide(x=w1047, y=3) -> (x/y=w1050:dbl)
                    n584 = To Word Integer(number=w1050) -> (16bit integer=w1049:i16)
                    n585 = Format Value(format string="%#g", value (0)=w1043) -> (output string=w1048:string)  [unwired: 1 in]
                    n586 = Replace Array Subset(array=w1051, new element=w1048, index (row)=w1049, index (col)=1) -> (w1046:string[][])
                  }
                  frame True {
                    n587 = local read "Re-Calculated Values Cluster"() -> (w1055:T9)
                    n588 = Unbundle By Name(w1055) -> ("Trap Density-VT"=w1054:dbl)
                    n589 = Search 1D Array(1D array=w1057, element="STS-Sat (V/decade):") -> (index of element=w1064:i32)  [unwired: 1 in]
                    n590 = Divide(x=w1064, y=3) -> (x/y=w1063:dbl)
                    n591 = To Word Integer(number=w1063) -> (16bit integer=w1065:i16)
                    n592 = Format Value(format string="%#g", value (0)=w1054) -> (output string=w1060:string)  [unwired: 1 in]
                    n593 = Build Array(w1056, w1060) -> (w1067:string[])
                    n594 = Increment(x=w1065) -> (x+1=w1066:i16)
                    n595 = Insert Into Array(array=w1058, index (row)=w1066, new element=w1067) -> (w1059:string[][])  [unwired: 1 in]
                  }
                }
                n596 = local write "Save Array"(w1039) -> ()
              }
              frame #13 {
                w1069 = "Trap Density-STS (Traps/Vcm^2):"
                n597 = local read "Save Array"() -> (w1071:string[][])
                n598 = Array Size(array=w1071) -> (size(s)=w1076:i32[])
                n599 = Array Subset(array=w1071, index (row)=0, index (col)=0, length (col)=3) -> (w1072:string[][])  [unwired: 1 in]
                n600 = Index Array(array=w1076, index=0) -> (element=w1078:i32)
                n601 = Reshape Array(w1072, w1078) -> (w1070:string[])
                n602 = Search 1D Array(1D array=w1070, element=w1069) -> (index of element=w1081:i32)  [unwired: 1 in]
                n603 = Equal?(x=w1081, y=-1) -> (x = y?=w1080:bool)
                n604 = case shown="True" w1080 {
                  tunnel: w1071 -> [w1091 w1098]
                  tunnel: w1081 -> [w1088 _]
                  tunnel: [w1087 w1099] -> w1079
                  tunnel: w1070 -> [_ w1097]
                  tunnel: w1069 -> [_ w1096]
                  frame False {
                    n605 = local read "Re-Calculated Values Cluster"() -> (w1084:T9)
                    n606 = Unbundle By Name(w1084) -> ("Trap Density-STS"=w1083:dbl)
                    n607 = Divide(x=w1088, y=3) -> (x/y=w1090:dbl)
                    n608 = To Word Integer(number=w1090) -> (16bit integer=w1089:i16)
                    n609 = Format Value(format string="%#g", value (0)=w1083) -> (output string=w1085:string)  [unwired: 1 in]
                    n610 = Replace Array Subset(array=w1091, new element=w1085, index (row)=w1089, index (col)=1) -> (w1087:string[][])
                  }
                  frame True {
                    n611 = local read "Re-Calculated Values Cluster"() -> (w1095:T9)
                    n612 = Unbundle By Name(w1095) -> ("Trap Density-STS"=w1094:dbl)
                    n613 = Search 1D Array(1D array=w1097, element="Trap Density-VT (Traps/Vcm^2):") -> (index of element=w1104:i32)  [unwired: 1 in]
                    n614 = Divide(x=w1104, y=3) -> (x/y=w1105:dbl)
                    n615 = To Word Integer(number=w1105) -> (16bit integer=w1103:i16)
                    n616 = Format Value(format string="%#g", value (0)=w1094) -> (output string=w1108:string)  [unwired: 1 in]
                    n617 = Build Array(w1096, w1108) -> (w1101:string[])
                    n618 = Increment(x=w1103) -> (x+1=w1102:i16)
                    n619 = Insert Into Array(array=w1098, index (row)=w1102, new element=w1101) -> (w1099:string[][])  [unwired: 1 in]
                  }
                }
                n620 = local write "Save Array"(w1079) -> ()
              }
            }
            n621 = local read "New: Temp"() -> (w616:dbl)
            n622 = local read "New: Width"() -> (w617:dbl)
            n623 = local read "New: Length"() -> (w619:dbl)
            n624 = local read "Index"() -> (w618:string)
            n625 = To Single Precision Float(number=w616) -> (single precision float=w633:sgl)
            n626 = Number To Decimal String(number=w633) -> (decimal integer string=w628:string)  [unwired: 1 in]
            n627 = To Single Precision Float(number=w617) -> (single precision float=w632:sgl)
            n628 = To Single Precision Float(number=w619) -> (single precision float=w631:sgl)
            n629 = Strip Path(path=w615) -> (stripped path=w620:path)  [unwired: 1 out]
            n630 = Number To Decimal String(number=w631) -> (decimal integer string=w626:string)  [unwired: 1 in]
            n631 = Number To Decimal String(number=w632) -> (decimal integer string=w625:string)  [unwired: 1 in]
            n632 = Concatenate Strings("_", w628, "K") -> (w630:string)
            n633 = call "Build Text"("Temp"=w630, "Index"=w618, "Length"=w626, "Width"=w625) -> ("Result"=w624:string)  [unwired: 10 in, 1 out]
            n634 = Path To String(path=w620) -> (string=w622:string)
            n635 = Concatenate Strings(w622, "\\", w624) -> (w623:string)
            n636 = String To Path(string=w623) -> (path=w614:path)
          }
          frame #1 {
            n637 = flat-sequence {
              tunnel: w1112 -> [w1114]
              tunnel: w1111 -> [w1113]
              tunnel: [w1113] -> w1110
              tunnel: w1110 -> [w1120]
              tunnel: w1109 -> [w1119]
              frame #0 {
                n638 = Equal?(x=w1114, y=w1113) -> (x = y?=w1115:bool)
                n639 = case shown="False" w1115 {
                  tunnel: w1114 -> [w1118 _]
                  tunnel: w1113 -> [w1117 _]
                  frame False {
                    n640 = Move(source path=w1118, 9:TRUE, 10:w1117) -> ()  [unwired: 2 in, 3 out]
                  }
                  frame True {
                  }
                }
              }
              frame #1 {
                n641 = local write "Transfer File"(w1120) -> ()
                n642 = call-poly <vilib>:"Write To Spreadsheet File.vi"("2D data"=w1119, "file path (dialog if empty)"=w1120) -> ()  [unwired: 6 in, 1 out]
              }
            }
          }
        }
        n643 = Cluster To Array(cluster=w604) -> (array=w603:bool[])
        n644 = Boolean Array To Number(Boolean array=w603) -> (number=w602:u32)
        n645 = Equal To 0?(x=w602) -> (x = 0?=w601:bool)
        n646 = case shown="True" w601 {
          tunnel: [MegaAwesome_States."Read Data" w608] -> w600
          tunnel: w599 -> [_ w612]
          frame False {
          }
          frame True {
            n647 = Unbundle By Name(w612) -> ("Save Next"=w611:bool)
            n648 = Select(t=MegaAwesome_States."No Event", s=w611, f=MegaAwesome_States."Next File") -> (s? t:f=w608:T2)
          }
        }
      }
      frame "Exit" {
      }
      frame "Save Lines" {
      }
      frame "Export" {
        n649 = flat-sequence {
          frame #0 {
            n650 = stacked-sequence {
              frame #0 {
                n651 = local read "Independant Variable:"() -> (w1127:string)
                n652 = Equal?(x=w1127, y="Length (um):") -> (x = y?=w1128:bool)
                n653 = case shown="True" w1128 {
                  frame False {
                  }
                  frame True {
                    n654 = local write "X Axis Display Type"("1") -> ()
                    n655 = local write "Opj X Axis"("2") -> ()
                  }
                }
              }
              frame #1 {
                n656 = local read "Independant Variable:"() -> (w1132:string)
                n657 = Equal?(x=w1132, y="Sample Temp (K):") -> (x = y?=w1133:bool)
                n658 = case shown="True" w1133 {
                  frame False {
                  }
                  frame True {
                    n659 = local write "X Axis Display Type"("1") -> ()
                    n660 = local write "Opj X Axis"("1") -> ()
                  }
                }
              }
              frame #2 {
                n661 = local read "Independant Variable:"() -> (w1137:string)
                n662 = Equal?(x=w1137, y="Mobility-Sat (cm^2/Vs):") -> (x = y?=w1138:bool)
                n663 = case shown="True" w1138 {
                  frame False {
                  }
                  frame True {
                    n664 = local write "X Axis Display Type"("2") -> ()
                    n665 = local write "Opj X Axis"("2") -> ()
                  }
                }
              }
              frame #3 {
                n666 = local read "Independant Variable:"() -> (w1142:string)
                n667 = Equal?(x=w1142, y="Mobility-Lin (cm^2/Vs):") -> (x = y?=w1143:bool)
                n668 = case shown="True" w1143 {
                  frame False {
                  }
                  frame True {
                    n669 = local write "X Axis Display Type"("2") -> ()
                    n670 = local write "Opj X Axis"("2") -> ()
                  }
                }
              }
              frame #4 {
                n671 = local read "Independant Variable:"() -> (w1147:string)
                n672 = Equal?(x=w1147, y="On/Off I-Sat:") -> (x = y?=w1148:bool)
                n673 = case shown="True" w1148 {
                  frame False {
                  }
                  frame True {
                    n674 = local write "X Axis Display Type"("2") -> ()
                    n675 = local write "Opj X Axis"("2") -> ()
                  }
                }
              }
              frame #5 {
                n676 = local read "Independant Variable:"() -> (w1152:string)
                n677 = Equal?(x=w1152, y="Off I-Sat (A):") -> (x = y?=w1153:bool)
                n678 = case shown="True" w1153 {
                  frame False {
                  }
                  frame True {
                    n679 = local write "X Axis Display Type"("2") -> ()
                    n680 = local write "Opj X Axis"("2") -> ()
                  }
                }
              }
              frame #6 {
                n681 = local read "Independant Variable:"() -> (w1157:string)
                n682 = Equal?(x=w1157, y="Vt-Sat (V):") -> (x = y?=w1158:bool)
                n683 = case shown="True" w1158 {
                  frame False {
                  }
                  frame True {
                    n684 = local write "X Axis Display Type"("1") -> ()
                    n685 = local write "Opj X Axis"("1") -> ()
                  }
                }
              }
              frame #7 {
                n686 = local read "Independant Variable:"() -> (w1162:string)
                n687 = Equal?(x=w1162, y="STS-Sat (V/decade):") -> (x = y?=w1163:bool)
                n688 = case shown="True" w1163 {
                  frame False {
                  }
                  frame True {
                    n689 = local write "X Axis Display Type"("1") -> ()
                    n690 = local write "Opj X Axis"("1") -> ()
                  }
                }
              }
              frame #8 {
                n691 = local read "Independant Variable:"() -> (w1167:string)
                n692 = Equal?(x=w1167, y="Trap Density-VT (Traps/Vcm^2):") -> (x = y?=w1168:bool)
                n693 = case shown="True" w1168 {
                  frame False {
                  }
                  frame True {
                    n694 = local write "X Axis Display Type"("2") -> ()
                    n695 = local write "Opj X Axis"("2") -> ()
                  }
                }
              }
              frame #9 {
                n696 = local read "Independant Variable:"() -> (w1172:string)
                n697 = Equal?(x=w1172, y="Trap Density-STS (Traps/Vcm^2):") -> (x = y?=w1173:bool)
                n698 = case shown="True" w1173 {
                  frame False {
                  }
                  frame True {
                    n699 = local write "X Axis Display Type"("2") -> ()
                    n700 = local write "Opj X Axis"("2") -> ()
                  }
                }
              }
            }
          }
          frame #1 {
            n701 = local read "Transfer Folder"() -> (w1181:path)
            n702 = Build Path(base path=w1181, name or relative path="Stats") -> (appended path=w1182:path)
            n703 = local read "Origin Project File"() -> (w1193:path)
            n704 = call <vilib>:"Check if File or Folder Exists.vi"("path"=w1182) -> ("file or folder exists?"=w1197:bool, "dup path"=w1196:path)  [unwired: 8 in, 1 out]
            n705 = call <userlib>:"OA_ConnectToOrigin.vi"() -> ("error out"=w1194:errorcluster, "Origin.IOApplication"=w1195:refnum<k7>)  [unwired: 8 in]
            n706 = case shown="False" w1197 {
              tunnel: w1196 -> [w1370 w1371]
              tunnel: [w1369 w1371] -> w1180
              frame False {
                n707 = Create Folder(path (use dialog)=w1370) -> (created path=w1369:path)  [unwired: 2 in, 2 out]
              }
              frame True {
              }
            }
            n708 = call "File Dialog"("start path"=w1182) -> ("selected path"=w1184:path)  [unwired: 11 in, 3 out]
            n709 = call <userlib>:"OA_Load.vi"("error in (no error)"=w1194, "Path"=w1193, "Origin.IOApplication"=w1195) -> ("error out"=w1191:errorcluster, "Origin.IOApplication"=w1192:refnum<k7>)  [unwired: 1 out]
            n710 = call "OAExecute.vi"("script"="document -m 3;", "Error IO"=w1191, "Origin.IOApplication"=w1192) -> ("Error IO Out"=w1189:errorcluster, "Origin.IOApplication"=w1190:refnum<k7>)  [unwired: 1 in, 1 out]
            n711 = local read "Independant Variable:"() -> (w1177:string)
            n712 = stacked-sequence {
              tunnel: w1181 -> [w1208 w1238 w1250 w1272 w1292 w1313 w1334 w1357]
              tunnel: w1180 -> [w1209 w1237 w1251 w1271 w1293 w1314 w1335 w1358]
              tunnel: w1190 -> [w1211 w1235 w1253 w1274 w1295 w1316 w1337 w1360]
              tunnel: w1189 -> [w1210 w1236 w1252 w1273 w1294 w1315 w1336 w1359]
              tunnel: [_ _ _ _ _ _ _ w1355] -> w1179
              tunnel: [_ _ _ _ _ _ _ w1356] -> w1178
              tunnel: w1177 -> [w1207 w1228 w1249 w1270 w1291 w1312 w1333 w1354]
              frame #0 {
                n713 = local read "X Axis Display Type"() -> (w1199:string)
                n714 = local read "Opj X Axis"() -> (w1204:string)
                n715 = Concatenate Strings("window -a MOBLGraph;\nlayer.x.type=", w1204, "; layer.x.label.numFormat = ", w1199, "; Y3 = 1; X3 = 1;", "window -a MOBLTable;\nwindow -s TV;") -> (w1202:string)
                n716 = call "Param_Analysis_7_24b_JW.vi"("Independant Variable"=w1207, "error in (no error)"=w1210, "Data Folder"=w1208, "Parameter String"="Mobility-Lin (cm^2/Vs):", "Parameter Name"="Mobility-Lin", "Stats Folder"=w1209) -> ("error out"=w1213:errorcluster, "Output Array"=w1215:string[][], "Variables"=w1206:T21)  [unwired: 2 in, 1 out]
                n717 = call "Origin_Export_7_27a_JW.vi"("Input Conditions"=w1206, "Analysis Array"=w1215, "error in (no error)"=w1213, "Parameter Worksheet Name"="[MOBLTable]Mobilities", "Parameter Folder Script"="pe_cd \"Mobility-Lin\";", "Origin.IOApplication"=w1211) -> ("error out"=w1212:errorcluster, "reference out"=w1214:refnum<k7>)  [unwired: 3 in, 1 out]
                n718 = call "OAExecute.vi"("script"=w1202, "Error IO"=w1212, "Origin.IOApplication"=w1214) -> ()  [unwired: 1 in, 3 out]
              }
              frame #1 {
                n719 = local read "X Axis Display Type"() -> (w1220:string)
                n720 = local read "Opj X Axis"() -> (w1225:string)
                n721 = Concatenate Strings("window -a MOBSGraph;\nlayer.x.type=", w1225, "; layer.x.label.numFormat = ", w1220, "; Y3 = 1; X3 = 1;", "window -a MOBSTable;\nwindow -s TV;") -> (w1223:string)
                n722 = call "Param_Analysis_7_24b_JW.vi"("Independant Variable"=w1228, "error in (no error)"=w1236, "Data Folder"=w1238, "Parameter String"="Mobility-Sat (cm^2/Vs):", "Parameter Name"="Mobility-Sat", "Stats Folder"=w1237) -> ("error out"=w1231:errorcluster, "Output Array"=w1229:string[][], "Variables"=w1227:T21)  [unwired: 2 in, 1 out]
                n723 = call "Origin_Export_7_27a_JW.vi"("Input Conditions"=w1227, "Analysis Array"=w1229, "error in (no error)"=w1231, "Parameter Worksheet Name"="[MOBSTable]Mobilities", "Parameter Folder Script"="pe_cd \"Mobility-Sat\";", "Origin.IOApplication"=w1235) -> ("error out"=w1230:errorcluster, "reference out"=w1232:refnum<k7>)  [unwired: 3 in, 1 out]
                n724 = call "OAExecute.vi"("script"=w1223, "Error IO"=w1230, "Origin.IOApplication"=w1232) -> ()  [unwired: 1 in, 3 out]
              }
              frame #2 {
                n725 = local read "X Axis Display Type"() -> (w1241:string)
                n726 = local read "Opj X Axis"() -> (w1246:string)
                n727 = Concatenate Strings("window -a NSTSGraph;\nlayer.x.type=", w1246, "; layer.x.label.numFormat = ", w1241, "; Y3 = 1; X3 = 1;", "window -a NSTSTable;\nwindow -s TV;") -> (w1244:string)
                n728 = call "Param_Analysis_7_24b_JW.vi"("Independant Variable"=w1249, "error in (no error)"=w1252, "Data Folder"=w1250, "Parameter String"="Trap Density-STS (Traps/Vcm^2):", "Parameter Name"="Trap Density-STS", "Stats Folder"=w1251) -> ("error out"=w1256:errorcluster, "Output Array"=w1254:string[][], "Variables"=w1248:T21)  [unwired: 2 in, 1 out]
                n729 = call "Origin_Export_7_27a_JW.vi"("Input Conditions"=w1248, "Analysis Array"=w1254, "error in (no error)"=w1256, "Parameter Worksheet Name"="[NSTSTable]Trap Densities", "Parameter Folder Script"="pe_cd \"N-STS\";", "Origin.IOApplication"=w1253) -> ("error out"=w1255:errorcluster, "reference out"=w1257:refnum<k7>)  [unwired: 3 in, 1 out]
                n730 = call "OAExecute.vi"("script"=w1244, "Error IO"=w1255, "Origin.IOApplication"=w1257) -> ()  [unwired: 1 in, 3 out]
              }
              frame #3 {
                n731 = local read "X Axis Display Type"() -> (w1262:string)
                n732 = local read "Opj X Axis"() -> (w1267:string)
                n733 = call "Param_Analysis_7_24b_JW.vi"("Independant Variable"=w1270, "error in (no error)"=w1273, "Data Folder"=w1272, "Parameter String"="Trap Density-VT (Traps/Vcm^2):", "Parameter Name"="Trap Density-Vt", "Stats Folder"=w1271) -> ("error out"=w1277:errorcluster, "Output Array"=w1275:string[][], "Variables"=w1269:T21)  [unwired: 2 in, 1 out]
                n734 = Concatenate Strings("window -a NVtGraph;\nlayer.x.type=", w1267, "; layer.x.label.numFormat = ", w1262, "; Y3 = 1; X3 = 1;", "window -a NVtTable;\nwindow -s TV;") -> (w1265:string)
                n735 = call "Origin_Export_7_27a_JW.vi"("Input Conditions"=w1269, "Analysis Array"=w1275, "error in (no error)"=w1277, "Parameter Worksheet Name"="[NVTTable]Trap Densities", "Parameter Folder Script"="pe_cd \"N-Vt\";", "Origin.IOApplication"=w1274) -> ("error out"=w1276:errorcluster, "reference out"=w1278:refnum<k7>)  [unwired: 3 in, 1 out]
                n736 = call "OAExecute.vi"("script"=w1265, "Error IO"=w1276, "Origin.IOApplication"=w1278) -> ()  [unwired: 1 in, 3 out]
              }
              frame #4 {
                n737 = local read "X Axis Display Type"() -> (w1283:string)
                n738 = local read "Opj X Axis"() -> (w1288:string)
                n739 = Concatenate Strings("window -a OffIGraph;\nlayer.x.type=", w1288, "; layer.x.label.numFormat = ", w1283, "; Y3 = 1; X3 = 1;", "window -a OffITable;\nwindow -s TV;") -> (w1286:string)
                n740 = call "Param_Analysis_7_24b_JW.vi"("Independant Variable"=w1291, "error in (no error)"=w1294, "Data Folder"=w1292, "Parameter String"="Off I-Sat (A):", "Parameter Name"="Off I-Sat", "Stats Folder"=w1293) -> ("error out"=w1298:errorcluster, "Output Array"=w1296:string[][], "Variables"=w1290:T21)  [unwired: 2 in, 1 out]
                n741 = call "Origin_Export_7_27a_JW.vi"("Input Conditions"=w1290, "Analysis Array"=w1296, "error in (no error)"=w1298, "Parameter Worksheet Name"="[OffItable]OffCurrents", "Parameter Folder Script"="pe_cd \"OffI-Sat\";", "Origin.IOApplication"=w1295) -> ("error out"=w1297:errorcluster, "reference out"=w1299:refnum<k7>)  [unwired: 3 in, 1 out]
                n742 = call "OAExecute.vi"("script"=w1286, "Error IO"=w1297, "Origin.IOApplication"=w1299) -> ()  [unwired: 1 in, 3 out]
              }
              frame #5 {
                n743 = local read "X Axis Display Type"() -> (w1304:string)
                n744 = local read "Opj X Axis"() -> (w1309:string)
                n745 = Concatenate Strings("window -a OnOffGraph;\nlayer.x.type=", w1309, "; layer.x.label.numFormat = ", w1304, "; Y3 = 1; X3 = 1;", "window -a OnOffTable;\nwindow -s TV;") -> (w1307:string)
                n746 = call "Param_Analysis_7_24b_JW.vi"("Independant Variable"=w1312, "error in (no error)"=w1315, "Data Folder"=w1313, "Parameter String"="On/Off I-Sat:", "Parameter Name"="OnOff Ratio", "Stats Folder"=w1314) -> ("error out"=w1319:errorcluster, "Output Array"=w1317:string[][], "Variables"=w1311:T21)  [unwired: 2 in, 1 out]
                n747 = call "Origin_Export_7_27a_JW.vi"("Input Conditions"=w1311, "Analysis Array"=w1317, "error in (no error)"=w1319, "Parameter Worksheet Name"="[OnOffTable]On/Off Ratios", "Parameter Folder Script"="pe_cd \"OnOff-Ratio\";", "Origin.IOApplication"=w1316) -> ("error out"=w1318:errorcluster, "reference out"=w1320:refnum<k7>)  [unwired: 3 in, 1 out]
                n748 = call "OAExecute.vi"("script"=w1307, "Error IO"=w1318, "Origin.IOApplication"=w1320) -> ()  [unwired: 1 in, 3 out]
              }
              frame #6 {
                n749 = local read "X Axis Display Type"() -> (w1325:string)
                n750 = local read "Opj X Axis"() -> (w1330:string)
                n751 = call "Param_Analysis_7_24b_JW.vi"("Independant Variable"=w1333, "error in (no error)"=w1336, "Data Folder"=w1334, "Parameter String"="STS-Sat (V/decade):", "Parameter Name"="STS-Sat", "Stats Folder"=w1335) -> ("error out"=w1340:errorcluster, "Output Array"=w1338:string[][], "Variables"=w1332:T21)  [unwired: 2 in, 1 out]
                n752 = Concatenate Strings("window -a SGraph;\nlayer.x.type=", w1330, "; layer.x.label.numFormat = ", w1325, "; Y3 = 1; X3 = 1;", "window -a STable;\nwindow -s TV;") -> (w1328:string)
                n753 = call "Origin_Export_7_27a_JW.vi"("Input Conditions"=w1332, "Analysis Array"=w1338, "error in (no error)"=w1340, "Parameter Worksheet Name"="[STable]Threshold Swing", "Parameter Folder Script"="pe_cd \"STS-Sat\";", "Origin.IOApplication"=w1337) -> ("error out"=w1339:errorcluster, "reference out"=w1341:refnum<k7>)  [unwired: 3 in, 1 out]
                n754 = call "OAExecute.vi"("script"=w1328, "Error IO"=w1339, "Origin.IOApplication"=w1341) -> ()  [unwired: 1 in, 3 out]
              }
              frame #7 {
                n755 = local read "X Axis Display Type"() -> (w1346:string)
                n756 = local read "Opj X Axis"() -> (w1351:string)
                n757 = Concatenate Strings("window -a VtGraph;\nlayer.x.type=", w1351, "; layer.x.label.numFormat = ", w1346, "; Y3 = 1; X3 = 1;", "window -a VtTable;\nwindow -s TV;") -> (w1349:string)
                n758 = call "Param_Analysis_7_24b_JW.vi"("Independant Variable"=w1354, "error in (no error)"=w1359, "Data Folder"=w1357, "Parameter String"="Vt-Sat (V):", "Parameter Name"="Vt-Sat", "Stats Folder"=w1358) -> ("error out"=w1363:errorcluster, "Output Array"=w1361:string[][], "Variables"=w1353:T21)  [unwired: 2 in, 1 out]
                n759 = call "Origin_Export_7_27a_JW.vi"("Input Conditions"=w1353, "Analysis Array"=w1361, "error in (no error)"=w1363, "Parameter Worksheet Name"="[VtTable]Threshold Voltages", "Parameter Folder Script"="pe_cd \"Vt-Sat\";", "Origin.IOApplication"=w1360) -> ("error out"=w1362:errorcluster, "reference out"=w1364:refnum<k7>)  [unwired: 3 in, 1 out]
                n760 = call "OAExecute.vi"("script"=w1349, "Error IO"=w1362, "Origin.IOApplication"=w1364) -> ("Error IO Out"=w1355:errorcluster, "Origin.IOApplication"=w1356:refnum<k7>)  [unwired: 1 in, 1 out]
              }
            }
            n761 = Path To String(path=w1184) -> (string=w1183:string)
            n762 = call "OAExecute.vi"("script"="pe_cd /; ", "Error IO"=w1179, "Origin.IOApplication"=w1178) -> ("Error IO Out"=w1185:errorcluster, "Origin.IOApplication"=w1186:refnum<k7>)  [unwired: 1 in, 1 out]
            n763 = call <userlib>:"OASaveProject.vi"("path"=w1183, "Error IO"=w1185, "Origin.IOApplication"=w1186) -> ()  [unwired: 3 out]
          }
        }
      }
    }
    "Current State" <- w14
    "Folder Index" <- w7
    n764 = Equal?(x=w16, y=MegaAwesome_States."Exit") -> (x = y?=w17:bool)
    n765 = Wait (ms)(milliseconds to wait=10) -> ()  [unwired: 1 out]
  }
